vi "RealTimeAcq_SynthFoc.vi"(4 "Frames/s":sgl=2.0, 5 "return to start":bool, 6 "Scan Axis":i8=3, 7 "Motion Board ID":T3=1 min=1 max=32 step=1, 8 "BKPT Shift":i32=75, 9 "mode":T1=enum."Full 25 Ch") -> (0 "error out":errorcluster, 2 "Bd ID Out":T2)   [LabVIEW 2022 SP3]
uses:
  ScanningControl/Motion Controllers/-MotionRoutines/MotionGlobals.vi
  <vilib>/Motion/FlexMotion/FunctionsVIs/Trajectory.llb/Load Acceleration/Deceleration.flx
  <vilib>/Motion/FlexMotion/CustomControls/CustomControls.llb/Axis To Control.flx
  <vilib>/Motion/FlexMotion/CustomControls/CustomControls.llb/Program.flx
  <instrlib>/niScope/Acquire/Fetch/niScope Multi Fetch Binary 8.vi
  <vilib>/Platform/TimedLoop/XDataNode/XDataNode.xnode
  <vilib>/Platform/TimedLoop/XDataNode/nitl_modes.ctl
  <vilib>/Platform/TimedLoop/XDataNode/XDNodeRunTimeDep.lvlib
  <vilib>/Platform/TimedLoop/XDataNode/wakeup.ctl
  <vilib>/Platform/TimedLoop/XDataNode/timing_clust.ctl
  <vilib>/Motion/FlexMotion/FunctionsVIs/Trajectory.llb/Wait for Move Complete (8 axes).flx
  <instrlib>/Acqiris Dx/Acqiris Dx.lvlib
  <vilib>/DAQmx/write.llb/DAQmx Write (Digital 1D Bool NChan 1Samp 1Line).vi
  Real Time/-RT_support/RealTimeMode.ctl
  Annular Array/-SynthApperture/TimeShiftDataI8.vi
  <vilib>/Analysis/NI_AALBase.lvlib
  <vilib>/Analysis/baseanly.llb/Mean (DBL).vi
panel:
  in  "Velocity Scale (%)":i16(slide) scale=50.0..110.0
  in  "Raw Name":string="raw"
  in  "Save Raw":bool
  in  "Type of Mean":u16(ring) items=["Mean from lines", "Mean just lines", "Poly Mean", "No mean"]
  out "Display queue":i32
  out "SF queue":i32
  out "Record queue":i32
  out "Display index":i32
  out "Read Loop":i32
  out "Read Data index":i32
  in  "Round to ROC?":bool
  in  "F3 20 MHz":dbl[](array[numeric])=[0.0, 0.0021173000000000003, 0.002217038688303391, 0.003063649156506908, 0.0031631091439381287, 0.0038030513383040436, 0.003902223261134889, 0.004435332245982045, 0.004534208485358321, 0.004999044189180914]
  in  "F2 40MHz":sgl[](array[numeric])=[0.0, 0.00132, 0.00142, 0.0019, 0.002, 0.00236, 0.00245, 0.00275, 0.00285, 0.0031]
  in  "One Way Receive":bool
  out "SF Index":i32
  in  "stop out":bool
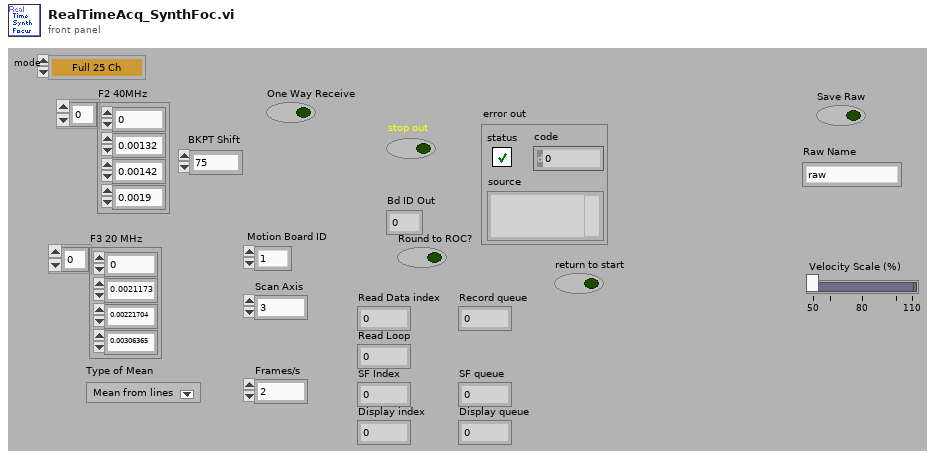
[diagram p1: front panel]
types:
  T1 = typedef "RealTimeMode.ctl" = enum16{"1T/5R", "1T/5R Deep Mem", "Full 25 Ch", "Drop Ch 5", "Drop Ch 5,4", "Drop Ch 5,4,3", "Drop Ch 5,4,3,2", "All 25 FIFO CH by CH", "Line by line 2 Ch", "Line by line All", "Deep Memory 2 CH", "Drop Ch 5 (3 Trig)", "test", "Drop Ch 5 XMIT", "Drop Ch 5,4 XMIT", "Drop Ch 5,4,3 XMIT"}
  T2 = typedef "Bd Id Out" = u8
  T3 = typedef "Board Id" = u8
  T4 = typedef "location.ctl" = enum16{"Automatic", "WCM Main", "Hawaii", "Columbia MM3000", "Columbia  NI System", "NYU", "RRI 2", "UHI Allen", "CUMC RT", "Chiba", "Stony Brook", "WCM Microscopy", "WCM Aeoretch", "WCM Optics Lab", "WCM Main 2Axis", "WCM Rotation", "WCM SAM SMAC", "SERI GP"}
  T5 = typedef "Program.flx" = u8
  T6 = typedef "XDNodeRunTimeDep.lvlib/timing_clust.ctl" = cluster{"Expected End [f-1]":u64, "Actual End [f-1]":u64, "Finished Late? [f-1]":bool, "Expected End [i-1]":u64, "Actual End [i-1]":u64, "Finished Late? [i-1]":bool, "Expected Start [i]":u64, "Actual Start [i]":u64, "Expected Start [f]":u64, "Actual Start [f]":u64, "Source Name":string, "Structure Name":string, "Period":i64, "Deadline":i64, "Offset":i64, "Start":i64, "Priority":i32, "Timeout":i32, "Mode":T7, "Wakeup Reason":T8, "Error":errorcluster, "Source Type":string, "Secondary Source Type":string, "Global End Time":u64, "Global Start Time":u64, "Frame Duration":u64, "Iteration Duration":u64, "Assigned CPU":i32, "I/O Scan Engine Mode":u32}
  T7 = typedef "XDNodeRunTimeDep.lvlib/nitl_modes.ctl" = enum32{"No Change", "Process missed periods, maintain original phase", "Discard missed periods, maintain original phase", "Process missed periods, ignore original phase", "Discard missed periods, ignore original phase"}
  T8 = typedef "XDNodeRunTimeDep.lvlib/wakeup.ctl" = enum32{"Normal", "Aborted", "Asynchronous wakeup", "Timing source error", "Timed loop error", "Timeout"}
  T9 = cluster{"gain":dbl, "wfm":i8[][], bool, "max queue size (-1, unlimited)":i32}
  T10 = typedef "Axis To Control.flx" = u16
  T11 = cluster{"ZoneStart":sgl[], "ZoneShift":sgl[], "ZoneLength":sgl[]}
  T12 = cluster{"ZoneStart":sgl[], "ZoneShift":sgl[], "ZoneLength":sgl[]}[][]
  T13 = cluster{"ZoneStart":sgl[], "ZoneShift":sgl[], "ZoneLength":sgl[]}[]
  T14 = cluster{"actualSamples":i32, "absoluteInitialX":dbl, "relativeInitialX":dbl, "xIncrement":dbl, "offset":dbl, "gain":dbl, "reserved1":dbl, "reserved2":dbl}[]
  T15 = cluster{"actualSamples":i32, "absoluteInitialX":dbl, "relativeInitialX":dbl, "xIncrement":dbl, "offset":dbl, "gain":dbl, "reserved1":dbl, "reserved2":dbl}
  T16 = cluster{"gain":dbl, "wfm":i8[][], "Reverse?":bool, i32}
  T17 = cluster{"dig gain":dbl, "Array":i8[][], "Reverse?":bool}
  T18 = typedef "Resource Out (Enum).flx" = u16
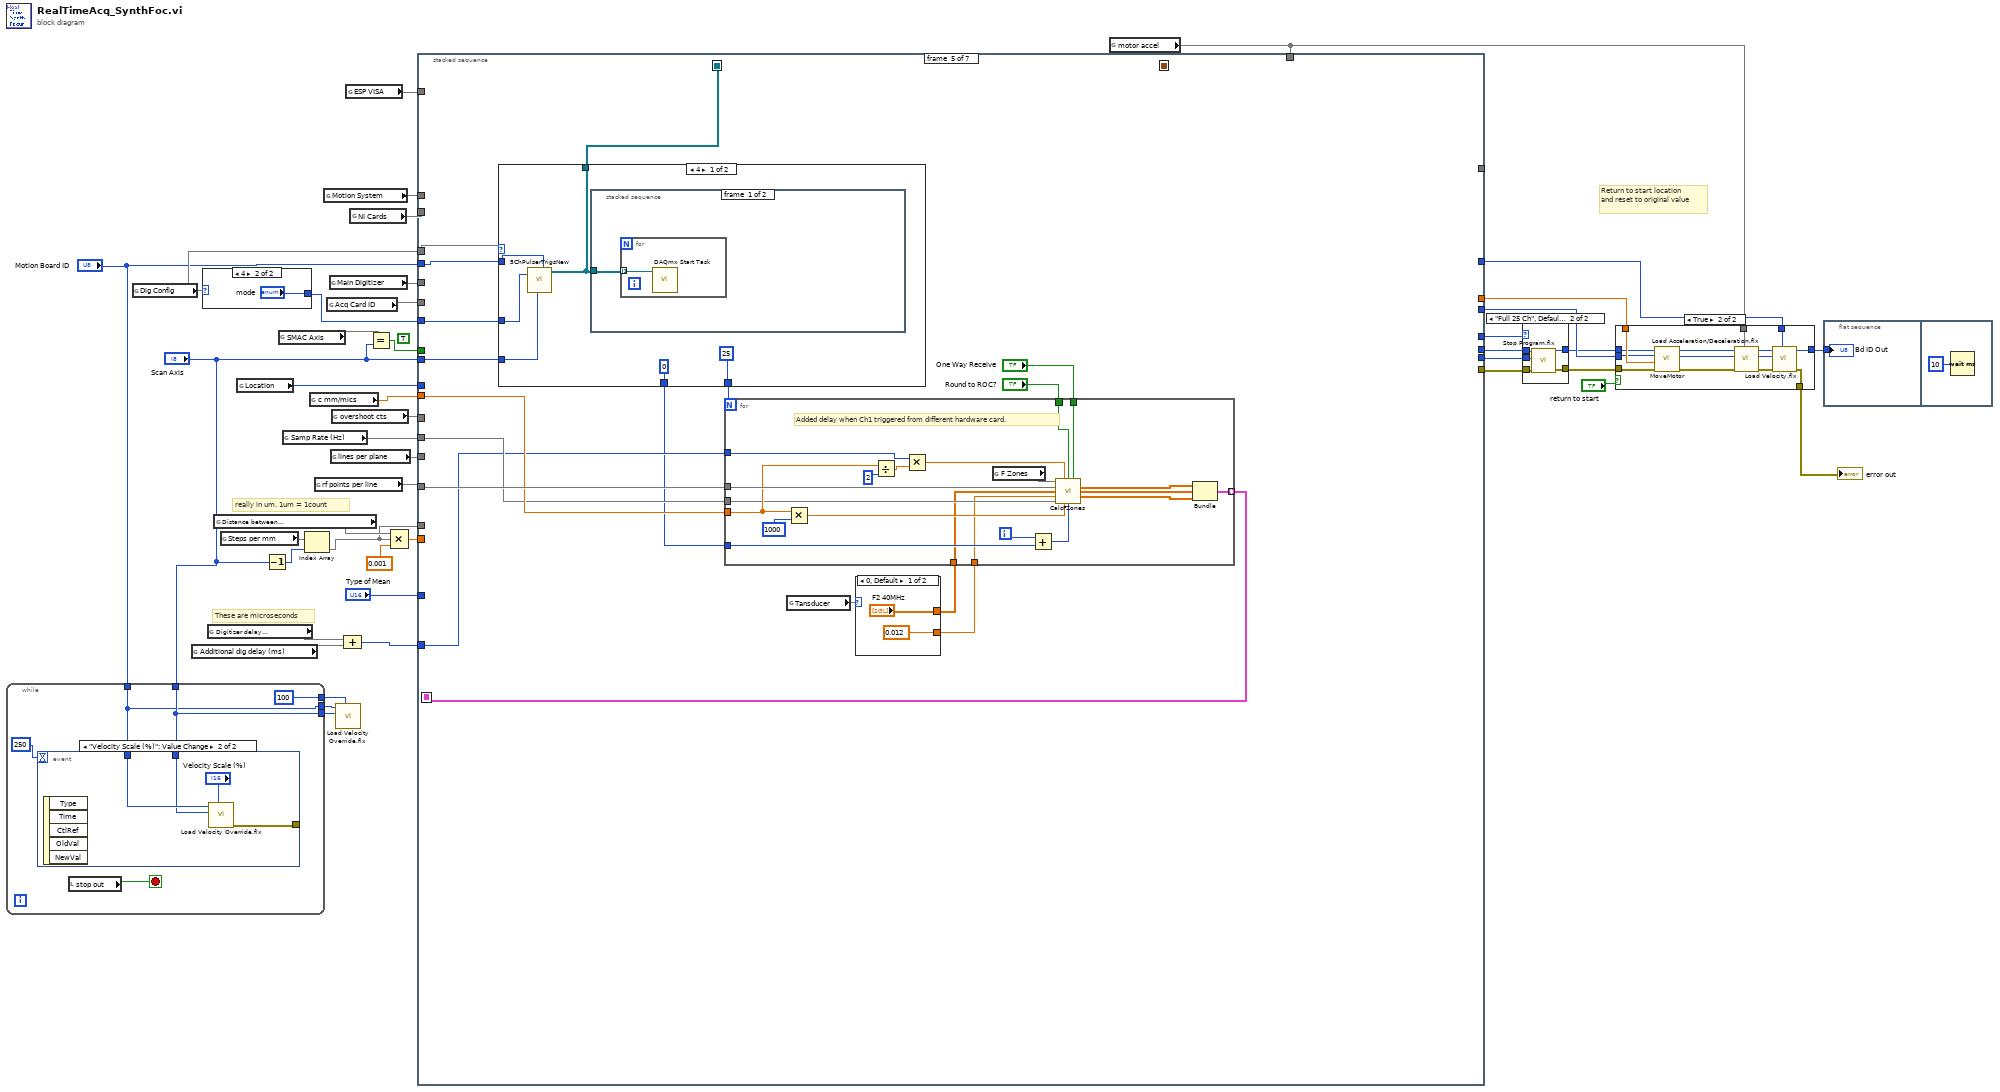
[diagram p0: block diagram]
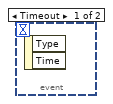
[diagram p2: hidden frame]
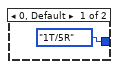
[diagram p3: hidden frame]
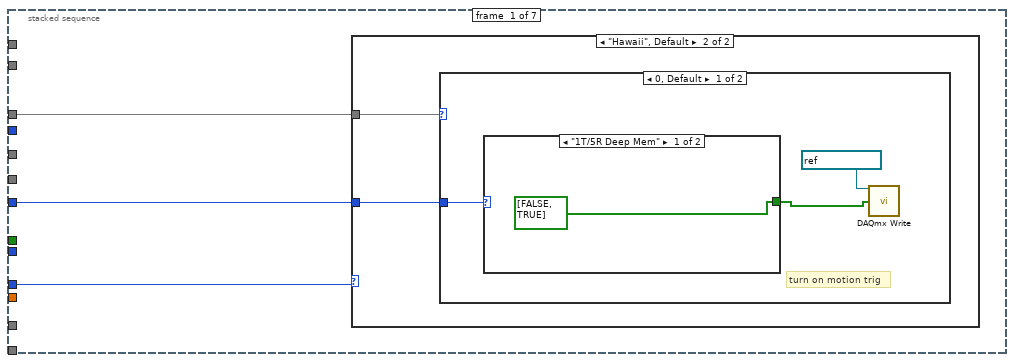
[diagram p6: hidden frame]
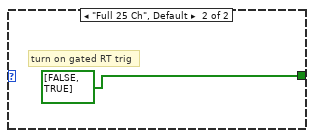
[diagram p8: hidden frame]
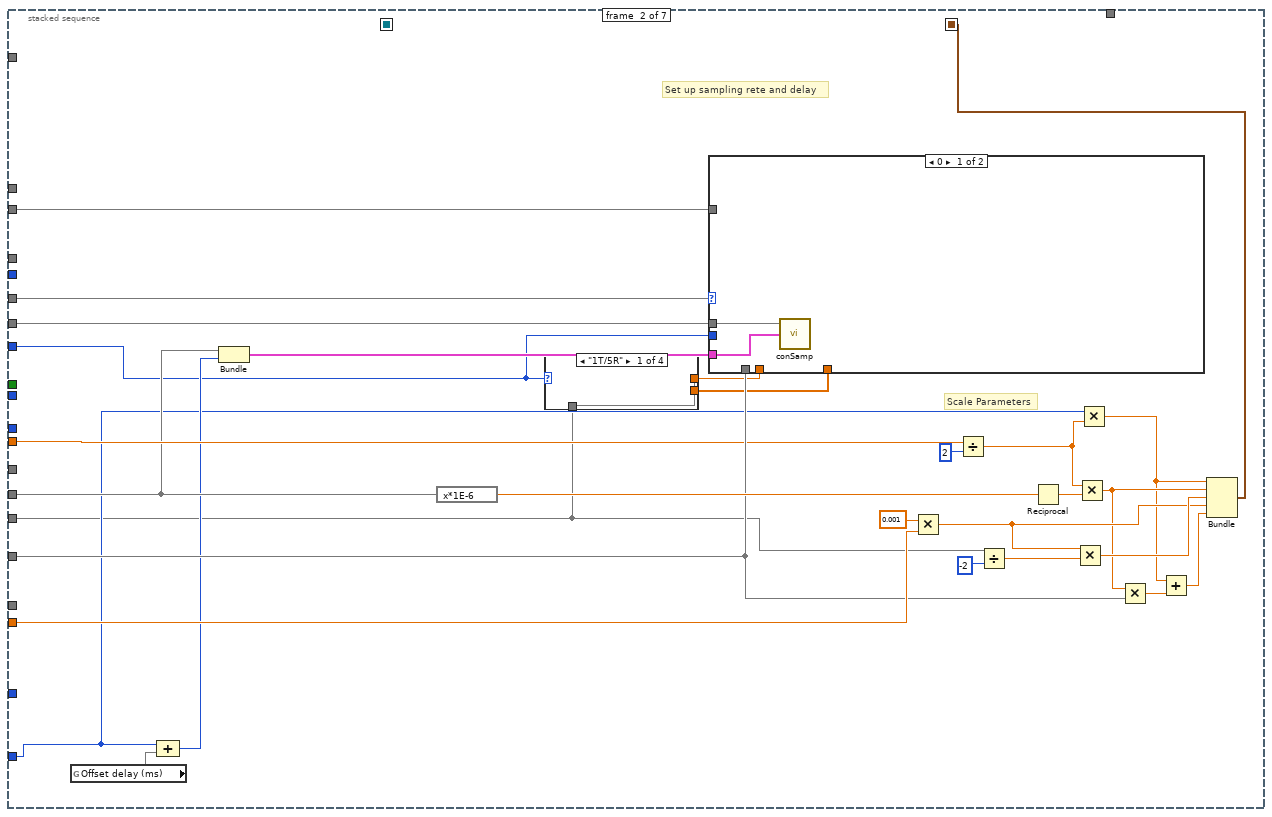
[diagram p10: hidden frame]
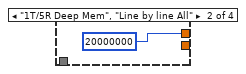
[diagram p11: hidden frame]
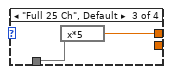
[diagram p12: hidden frame]
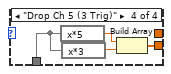
[diagram p13: hidden frame]
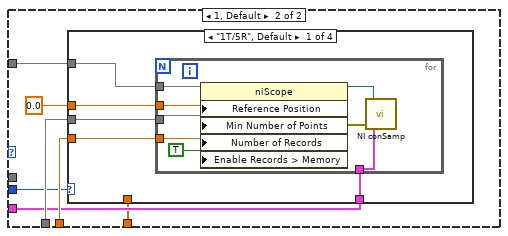
[diagram p14: hidden frame]
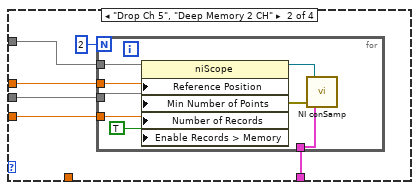
[diagram p15: hidden frame]
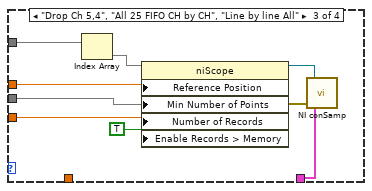
[diagram p16: hidden frame]
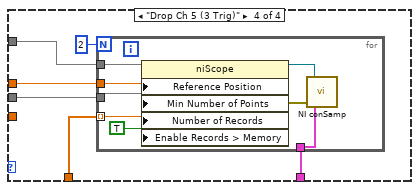
[diagram p17: hidden frame]
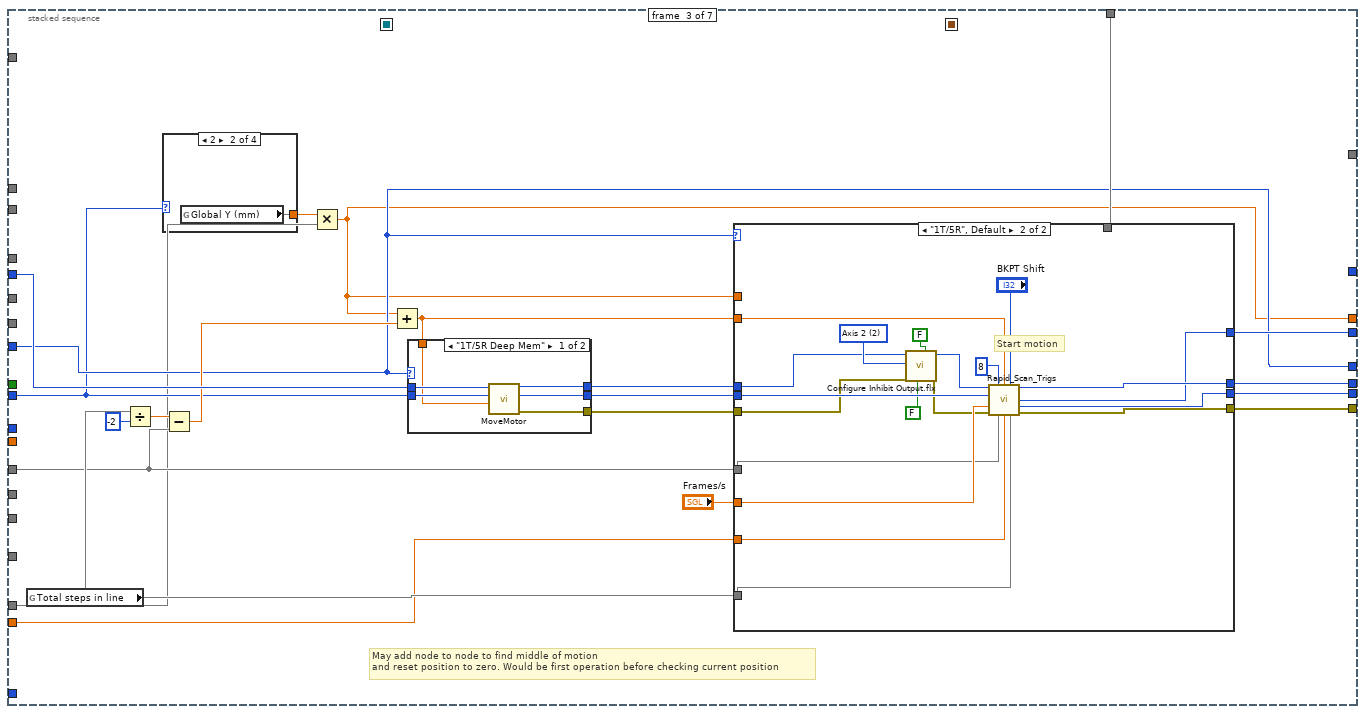
[diagram p18: hidden frame]
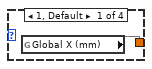
[diagram p19: hidden frame]
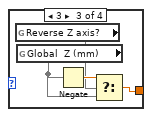
[diagram p20: hidden frame]
diagram:
  (unwired) TRUE
  # "These are microseconds"
  # "really in um. 1um = 1count"
  # "Return to start location and reset to original value"
  n1 = while {
    tunnel: "Motion Board ID" -> [w44]
    tunnel: "Scan Axis" -> [w45]
    tunnel: [100] -> w6
    tunnel: [w45] -> w5
    tunnel: [w44] -> w4
    stop <- w48 stop-if-true
    n2 = event shown="[1] \"Velocity Scale (%)\": Value Change" {
      selector: _ -> [_ _]
      dyn-events: _ -> [_ _]
      timeout: 250 -> [_ _]
      tunnel: w44 -> [_ w51]
      tunnel: w45 -> [_ w50]
      tunnel: [_ w49] -> _
      event Timeout {
        n3 = event-data() -> ()  [unwired: 1 in, 2 out]
      }
      event "Velocity Scale (%)": Value Change {
        n4 = event-data() -> ()  [unwired: 1 in, 5 out]
        n5 = call <vilib>:"Load Velocity Override.flx"("Override  Percentage (100%)"="Velocity Scale (%)", "Axis or Vector Space"=w50, "Board ID"=w51) -> ("error out"=w49:errorcluster)  [unwired: 4 in, 2 out]
      }
    }
    n6 = local read "stop out"() -> (w48:bool)
  }
  n7 = global read "MotionGlobals.vi" "Dig Config"() -> (w13)
  n8 = global read "MotionGlobals.vi" "Additional dig delay (ms)"() -> (w24)
  n9 = case shown="4" w13 {
    tunnel: [RealTimeMode."1T/5R" ("mode 2") "mode"] -> w15
    frame 0, Default {
    }
    frame 4 {
    }
  }
  n10 = global read "MotionGlobals.vi" "Digitizer delay\n (ms)"() -> (w25)
  n11 = global read "MotionGlobals.vi" "Distance between\nscan lines (mm)"() -> (w33)
  n12 = global read "MotionGlobals.vi" "Steps per mm"() -> (w12)
  n13 = global read "MotionGlobals.vi" "Location"() -> (w2:T4)
  n14 = Decrement(x="Scan Axis") -> (x-1=w11:i8)
  n15 = global read "MotionGlobals.vi" "SMAC Axis"() -> (w1)
  n16 = global read "MotionGlobals.vi" "Samp Rate (Hz)"() -> (w22)
  n17 = Index Array(array=w12, index=w11) -> (element=w10)
  n18 = global read "MotionGlobals.vi" "c mm/mics"() -> (w26:sgl)
  n19 = global read "MotionGlobals.vi" "rf points per line"() -> (w42)
  n20 = global read "MotionGlobals.vi" "Motion System"() -> (w9)
  n21 = global read "MotionGlobals.vi" "Acq Card ID"() -> (w30)
  n22 = global read "MotionGlobals.vi" "Main Digitizer"() -> (w31)
  n23 = global read "MotionGlobals.vi" "lines per plane"() -> (w43)
  n24 = global read "MotionGlobals.vi" "overshoot cts"() -> (w41)
  n25 = call <vilib>:"Load Velocity Override.flx"("Override  Percentage (100%)"=w6, "Axis or Vector Space"=w5, "Board ID"=w4) -> ()  [unwired: 4 in, 3 out]
  n26 = Compound Arithmetic op=ADD(w25, w24) -> (w23:i32)
  n27 = global read "MotionGlobals.vi" "ESP VISA"() -> (w16)
  n28 = global read "MotionGlobals.vi" "NI Cards"() -> (w3)
  n29 = Equal?(x=w1, y="Scan Axis") -> (x = y?=w21:bool)
  n30 = Compound Arithmetic op=MULTIPLY(w33, w10, 0.001) -> (w32:dbl)
  n31 = global read "MotionGlobals.vi" "motor accel"() -> (w28)
  n32 = stacked-sequence {
    seq-local: [_ w85 _ _ _ _ _] -> [_ _ _ _ _ w299 _]
    seq-local: [_ _ _ _ w242 _ _] -> [_ _ _ _ _ w298 _]
    seq-local: [_ _ _ _ w239 _ _] -> [_ _ _ _ _ _ w2097]
    tunnel: w30 -> [_ w92 _ _ _ w306 _]
    tunnel: w43 -> [_ w67 _ _ _ w305 _]
    tunnel: [_ _ w181 _ _ _ _] -> w37
    tunnel: [_ _ w180 _ _ _ _] -> w39
    tunnel: w42 -> [_ w75 _ _ w248 w304 _]
    tunnel: [_ _ w178 _ _ _ _] -> w38
    tunnel: [_ _ w165 _ _ _ _] -> w36
    tunnel: w41 -> [_ _ w174 _ _ _ _]
    tunnel: [_ _ w177 _ _ _ _] -> w40
    tunnel: "Motion Board ID" -> [_ _ w173 w229 w238 w303 _]
    tunnel: [_ _ w168 _ _ _ _] -> w35
    tunnel: w15 -> [w56 w66 w168 _ w236 w295 _]
    tunnel: "Scan Axis" -> [_ _ w167 _ w232 w296 _]
    tunnel: w32 -> [_ w78 w172 _ _ _ _]
    tunnel: w31 -> [_ w77 _ _ _ w302 _]
    tunnel: [_ _ _ _ _ w301 _] -> w29
    tunnel: w28 -> [_ _ w170 _ _ _ _]
    tunnel: w9 -> [_ _ _ w230 _ w300 _]
    tunnel: [_ _ _ _ _ w300 _] -> _
    tunnel: w2 -> [w57 _ _ _ _ _ w2099]
    tunnel: w26 -> [_ w74 _ _ w247 _ _]
    tunnel: w23 -> [_ w70 _ _ w245 _ _]
    tunnel: w22 -> [_ w73 _ _ w246 _ _]
    tunnel: w21 -> [_ _ _ _ _ w294 _]
    tunnel: w3 -> [_ w69 _ _ _ w297 _]
    tunnel: w16 -> [_ _ _ _ _ _ _]
    tunnel: "Type of Mean" -> [_ _ _ _ _ w293 _]
    tunnel: w13 -> [w55 _ _ _ w237 _ w2095]
    tunnel: w10 -> [_ _ w164 _ _ _ _]
    frame #0 {
      n33 = case shown="\"Hawaii\", Default" w57 {
        tunnel: w56 -> [_ w59]
        tunnel: w55 -> [_ w58]
        frame "UHI Allen", "CUMC RT" {
        }
        frame "Hawaii", Default {
          n34 = case shown="0, Default" w58 {
            tunnel: w59 -> [w62 _]
            frame 0, Default {
              # "turn on motion trig"
              n35 = case shown="\"1T/5R Deep Mem\"" w62 {
                tunnel: [bool[] [FALSE, TRUE] ("data") bool[] [FALSE, TRUE] ("data")] -> w60
                frame "1T/5R Deep Mem" {
                }
                frame "Full 25 Ch", Default {
                  # "turn on gated RT trig"
                }
              }
              n36 = call-poly <vilib>:"DAQmx Write.vi"("task/channels in"=refnum<k21> "DIO-L2 L3", "data"=w60) -> ()  [unwired: 11 in, 3 out]
            }
            frame 4 {
            }
          }
        }
      }
    }
    frame #1 {
      # "Scale Parameters"
      # "Set up sampling rete and delay"
      n37 = global read "MotionGlobals.vi" "Offset delay (ms)"() -> (w72)
      n38 = Compound Arithmetic op=ADD(w70, w72) -> (w71:i32)
      n39 = Bundle("Samp Rate (Hz)"=w73, w71) -> (w93:cluster{"Samp Rate (Hz)":void, i32})  [unwired: 1 out]
      n40 = expression code="x*1E-6"(w73) -> (w76:dbl)
      n41 = case shown="\"1T/5R\"" w66 {
        tunnel: [w94 20000000 w96 _] -> w68
        tunnel: w67 -> [w94 _ w97 w101]
        tunnel: [_ _ _ w98] -> w65
        frame "1T/5R" {
        }
        frame "1T/5R Deep Mem", "Line by line All" {
        }
        frame "Full 25 Ch", Default {
          n42 = expression code="x*5"(w97) -> (w96:dbl)
        }
        frame "Drop Ch 5 (3 Trig)" {
          n43 = expression code="x*5"(w101) -> (w100:dbl)
          n44 = expression code="x*3"(w101) -> (w99:dbl)
          n45 = Build Array(w100, w99) -> (w98:dbl[])
        }
      }
      n46 = case shown="0" w77 {
        tunnel: w93 -> [w103 w108]
        tunnel: w92 -> [w102 _]
        tunnel: w75 -> [_ w109]
        tunnel: w68 -> [_ w110]
        tunnel: w69 -> [_ w107]
        tunnel: w66 -> [_ w105]
        tunnel: w65 -> [_ w104]
        frame 0 {
          n47 = call "conSamp.vi"("Sampling"=w103, "InstrumentID"=w102) -> ()  [unwired: 1 in, 2 out]
        }
        frame 1, Default {
          n48 = case shown="\"1T/5R\", Default" w105 {
            tunnel: w110 -> [w115 w129 w146 _]
            tunnel: w109 -> [w114 w128 w145 w152]
            tunnel: w108 -> [w113 w127 w144 w151]
            tunnel: w107 -> [w112 w126 w142 w150]
            tunnel: 0.0 -> [w111 w125 w143 w149]
            tunnel: w104 -> [_ _ _ w147]
            frame "1T/5R", Default {
              n49 = for {
                tunnel: w115 -> [w118]
                tunnel: w114 -> [w123]
                tunnel: w112 -> [w120]
                tunnel: w113 -> [w119]
                tunnel: w111 -> [w117]
                n50 = property class="niScope"(reference=w120, "Reference Position"=w117, "Min Number of Points"=w123, "Number of Records"=w118, "Enable Records > Memory"=TRUE) -> (reference out=w122:refnum<k15>, error out=w121:errorcluster)  [unwired: 1 in]
                n51 = call "NI conSamp.vi"("error in"=w121, "Sampling"=w119, "InstrumentID"=w122) -> ()  [unwired: 2 out]
              }
            }
            frame "Drop Ch 5", "Deep Memory 2 CH" {
              n52 = for {
                N: 2 -> [_]
                tunnel: w129 -> [w132]
                tunnel: w128 -> [w137]
                tunnel: w126 -> [w134]
                tunnel: w127 -> [w133]
                tunnel: w125 -> [w131]
                n53 = property class="niScope"(reference=w134, "Reference Position"=w131, "Min Number of Points"=w137, "Number of Records"=w132, "Enable Records > Memory"=TRUE) -> (reference out=w136:refnum<k15>, error out=w135:errorcluster)  [unwired: 1 in]
                n54 = call "NI conSamp.vi"("error in"=w135, "Sampling"=w133, "InstrumentID"=w136) -> ()  [unwired: 2 out]
              }
            }
            frame "Drop Ch 5,4", "All 25 FIFO CH by CH", "Line by line All" {
              n55 = Index Array(array=w142) -> (element=w138)  [unwired: 1 in]
              n56 = property class="niScope"(reference=w138, "Reference Position"=w143, "Min Number of Points"=w145, "Number of Records"=w146, "Enable Records > Memory"=TRUE) -> (reference out=w141:refnum<k15>, error out=w140:errorcluster)  [unwired: 1 in]
              n57 = call "NI conSamp.vi"("error in"=w140, "Sampling"=w144, "InstrumentID"=w141) -> ()  [unwired: 2 out]
            }
            frame "Drop Ch 5 (3 Trig)" {
              n58 = for {
                N: 2 -> [_]
                tunnel: w147 -> [w155] mode=indexing
                tunnel: w152 -> [w160]
                tunnel: w150 -> [w157]
                tunnel: w151 -> [w156]
                tunnel: w149 -> [w154]
                n59 = property class="niScope"(reference=w157, "Reference Position"=w154, "Min Number of Points"=w160, "Number of Records"=w155, "Enable Records > Memory"=TRUE) -> (reference out=w159:refnum<k15>, error out=w158:errorcluster)  [unwired: 1 in]
                n60 = call "NI conSamp.vi"("error in"=w158, "Sampling"=w156, "InstrumentID"=w159) -> ()  [unwired: 2 out]
              }
            }
          }
        }
      }
      n61 = Multiply(x=0.001, y=w78) -> (x*y=w83:dbl)
      n62 = Divide(x=w74, y=2) -> (x/y=w86:sgl)
      n63 = Divide(x=w67, y=-2) -> (x/y=w88:dbl)
      n64 = Reciprocal(x=w76) -> (1/x=w91:dbl)
      n65 = Multiply(x=w83, y=w88) -> (x*y=w84:dbl)
      n66 = Multiply(x=w86, y=w91) -> (x*y=w82:dbl)
      n67 = Multiply(x=w70, y=w86) -> (x*y=w80:sgl)
      n68 = Multiply(x=w82, y=w75) -> (x*y=w81:dbl)
      n69 = Add(x=w80, y=w81) -> (x+y=w79:sgl)
      n70 = Bundle(w80, w82, w84, w83, w79) -> (w85:cluster{sgl, dbl, dbl, dbl, sgl})  [unwired: 1 out]
    }
    frame #2 {
      # "May add node to node to find middle of motion\nand reset position to zero. Would be first operation before checking current position"
      n71 = global read "MotionGlobals.vi" "Total steps in line"() -> (w176)
      n72 = Divide(x=w176, y=-2) -> (x/y=w175:dbl)
      n73 = case shown="2" w167 {
        tunnel: [w183 w184 w185 w189] -> w166
        frame 1, Default {
          n74 = global read "MotionGlobals.vi" "Global X (mm)"() -> (w183)
        }
        frame 2 {
          n75 = global read "MotionGlobals.vi" "Global Y (mm)"() -> (w184)
        }
        frame 3 {
          n76 = global read "MotionGlobals.vi" "Reverse Z axis?"() -> (w186)
          n77 = global read "MotionGlobals.vi" "Global  Z (mm)"() -> (w187)
          n78 = Negate(x=w187) -> (-x=w188:dbl)
          n79 = Select(t=w188, s=w186, f=w187) -> (s? t:f=w185:dbl)
        }
        frame 4 {
          n80 = global read "MotionGlobals.vi" "Global  Axis 4"() -> (w189)
        }
      }
      n81 = Subtract(x=w175, y=w174) -> (x-y=w171:dbl)
      n82 = Multiply(x=w166, y=w164) -> (x*y=w165:dbl)
      n83 = Add(x=w165, y=w171) -> (x+y=w169:dbl)
      n84 = case shown="\"1T/5R Deep Mem\"" w168 {
        tunnel: w173 -> [w195 w197]
        tunnel: w167 -> [w194 w196]
        tunnel: [w193 w197] -> w161
        tunnel: [w192 w196] -> w163
        tunnel: [w191 _] -> w162
        tunnel: w169 -> [w190 _]
        frame "1T/5R Deep Mem" {
          n85 = call "MoveMotor.vi"("Target Position (0)"=w190, "Axis or Vector Space"=w194, "Motion Bd ID"=w195) -> ("error out"=w191:errorcluster, "Resource Output"=w192:u16, "Bd ID Out"=w193:u8)  [unwired: 2 in, 4 out]
        }
        frame "Full 25 Ch", Default {
        }
      }
      n86 = case shown="\"1T/5R\", Default" w168 {
        tunnel: "Frames/s" -> [w207 w228]
        tunnel: [w198 w227] -> w181
        tunnel: [w209 w226] -> w180
        tunnel: [_ w225] -> w178
        tunnel: [w208 w224] -> w177
        tunnel: w176 -> [w205 w223]
        tunnel: w172 -> [_ w222]
        tunnel: w174 -> [_ w221]
        tunnel: w161 -> [w209 w211]
        tunnel: w163 -> [w208 w220]
        tunnel: w162 -> [w199 w210]
        tunnel: w169 -> [_ w219]
        tunnel: w165 -> [w206 _]
        tunnel: w170 -> [_ _]
        frame "1T/5R Deep Mem", "Line by line All" {
          w201 = T5 6 ("Program (1)")
          w204 = FALSE
          n87 = call "Modulo_Triggers.vi"("Motion Settings In"=w209, "Axis"=w208, "Reverse ?"=w204, "Program (1)"=w201, 7:w207, "error in (no error)"=w199, 12:w205, "Offset"=w206) -> ("error out"=w200:errorcluster)  [unwired: 1 in, 6 out]
          n88 = Increment(x=w201) -> (x+1=w202:T5)
          n89 = Not(x=w204) -> (.not. x?=w203:bool)
          n90 = call "Modulo_Triggers.vi"("Motion Settings In"=w209, "Axis"=w208, "Reverse ?"=w203, "Program (1)"=w202, 7:w207, "error in (no error)"=w200, 12:w205, "Offset"=w206) -> ("error out"=w198:errorcluster)  [unwired: 1 in, 6 out]
        }
        frame "1T/5R", Default {
          w214 = T10 2 items=["Axis 1"=1, "Axis 2"=2, "Axis 3"=3, "Axis 4"=4, "Axis 5"=5, "Axis 6"=6, "Axis 7"=7, "Axis 8"=8] ("Axis")
          # "Start motion"
          n91 = call <vilib>:"Configure Inhibit Output.flx"("Enable"=FALSE, "Polarity (Active Low)"=FALSE, "error in (no error)"=w210, "Axis"=w214, "Board ID"=w211) -> ("error out"=w217:errorcluster, "Bd ID Out"=w218:T2)  [unwired: 1 in, 4 out]
          n92 = call "Rapid_Scan_Trigs.vi"("Board ID"=w218, "Program (1)"=T5 8, "Start Position"=w219, "BKPT Shift"="BKPT Shift", "Scan Axis"=w220, "# frames/ s"=w228, "error in (no error)"=w217, "overshoot"=w221, "step interval"=w222, "Total Steps (one way)"=w223) -> ("Bd ID Out"=w226:u8, "Axis Resource out"=w224:u16, "Program ID"=w225:u8, "error out"=w227:errorcluster)  [unwired: 1 in, 1 out]
        }
      }
    }
    frame #3 {
      n93 = case shown="0, Default" w230 {
        tunnel: w229 -> [w231 _]
        frame 0, Default {
          n94 = call "CheckLimStat.vi"("Motion Board ID"=w231) -> ()
        }
        frame 1, 7 {
        }
      }
    }
    frame #4 {
      n95 = case shown="4" w237 {
        tunnel: [25 5] -> w241
        tunnel: [u32 0 w267] -> w240
        tunnel: [w253 _] -> w239
        tunnel: w238 -> [w256 _]
        tunnel: w236 -> [w255 _]
        tunnel: w232 -> [w254 _]
        frame 4 {
          n96 = call "5ChPulserTrigsNew.vi"("Motion Settings"=w256, "Digitizer Settings"=w255, "Axis"=w254) -> ("5CH Pulser Tasks"=w253:refnum<k21>[])  [unwired: 6 in, 1 out]
          n97 = stacked-sequence {
            tunnel: w253 -> [w259 _]
            frame #0 {
              n98 = for {
                tunnel: w259 -> [w260] mode=indexing
                n99 = call <vilib>:"DAQmx Start Task.vi"("task/channels in"=w260) -> ()  [unwired: 1 in, 14 out]
              }
            }
            frame #1 {
              n100 = for {
                tunnel: bool[][] [[TRUE], [FALSE]] ("data") -> [w262] mode=indexing
                n101 = flat-sequence {
                  tunnel: w262 -> [w265]
                  tunnel: [w265] -> w263
                  tunnel: w263 -> [w266]
                  frame #0 {
                    n102 = Wait (ms)(milliseconds to wait=u32 25) -> ()  [unwired: 1 out]
                  }
                  frame #1 {
                    n103 = call "DAQ Assistant"("data"=w266) -> ()  [unwired: 17 in, 2 out]
                  }
                }
              }
            }
          }
        }
        frame 0, Default {
          n104 = global read "MotionGlobals.vi" "Switch T/R"() -> (w270)
          n105 = Decrement(x=w270) -> (x-1=w269:dbl)
          n106 = Multiply(x=w269, y=5) -> (x*y=w267:i32)
        }
      }
      n107 = global read "MotionGlobals.vi" "Tansducer"() -> (w235)
      n108 = case shown="0, Default" w235 {
        tunnel: ["F2 40MHz" "F3 20 MHz"] -> w234
        tunnel: [0.012 ("ROC (mm)") 0.031 ("ROC (mm)")] -> w233
        frame 0, Default {
        }
        frame 1 {
        }
      }
      n109 = for {
        N: w241 -> [_]
        tunnel: w248 -> [w288]
        tunnel: w247 -> [w281]
        tunnel: w246 -> [w276]
        tunnel: w245 -> [w287]
        tunnel: "One Way Receive" -> [w286]
        tunnel: "Round to ROC?" -> [w285]
        tunnel: [w283] -> w242 mode=indexing
        tunnel: w240 -> [w278]
        tunnel: w234 -> [w273]
        tunnel: w233 -> [w272]
        i -> [w277]
        # "Added delay when Ch1 triggered from different hardware card."
        n110 = Multiply(x=w281, y=1000) -> (x*y=w282:sgl)
        n111 = Divide(x=w281, y=2) -> (x/y=w291:sgl)
        n112 = Multiply(x=w287, y=w291) -> (x*y=w280:sgl)
        n113 = global read "MotionGlobals.vi" "F Zones"() -> (w290)
        n114 = Add(x=w277, y=w278) -> (x+y=w279:u32)
        n115 = call "CalcFZones.vi"("F- zones"=w290, "delay (mm)"=w280, "Round to ROC?"=w285, "One Way Receive"=w286, "# rf points per line"=w288, "Radii (m)"=w273, "ROC (m)"=w272, "Sampling Rate"=w276, "c (m/s)"=w282, "File index number"=w279) -> ("ZoneStart"=w275:sgl[], "ZoneShift"=w274:sgl[], "ZoneLength"=w284:sgl[])  [unwired: 3 out]
        n116 = Bundle("ZoneStart"=w275, "ZoneShift"=w274, "ZoneLength"=w284) -> (w283:T11)  [unwired: 1 in]
      }
    }
    frame #5 {
      n117 = case shown="True" w294 {
        tunnel: w306 -> [w315 _]
        tunnel: w305 -> [w316 w408]
        tunnel: w304 -> [w317 w407]
        tunnel: w303 -> [w313 w409]
        tunnel: w299 -> [w312 w406]
        tunnel: w302 -> [w311 _]
        tunnel: [w310 w410] -> w301
        tunnel: w300 -> [w309 _]
        tunnel: w298 -> [_ w405]
        tunnel: w295 -> [_ w404]
        tunnel: w297 -> [w308 w403]
        tunnel: w296 -> [_ w402]
        tunnel: w293 -> [_ w401]
        frame False {
          n118 = Index Array(array=w308) -> (element=w307)  [unwired: 1 in]
          n119 = while {
            tunnel: w317 -> [w339]
            tunnel: w316 -> [w329]
            tunnel: w315 -> [w338]
            shift-right: [w337] -> _
            shift-left: TRUE -> [w322]
            tunnel: w313 -> [w336]
            tunnel: w312 -> [w332]
            tunnel: w311 -> [w330]
            tunnel: w309 -> [w323]
            tunnel: w307 -> [w318]
            i -> [w331]
            stop <- w335 stop-if-true
            # "Display data"
            # "Get data"
            # "This is slower version for heavier mass motors. Scan stop, read data, scan etc"
            n120 = Select(t="1", s=w322, f="2") -> (s? t:f=w319:string)
            n121 = Select(t=T5 6 ("Program (1)"), s=w322, f=T5 7 ("Program (1)")) -> (s? t:f=w326:T5)
            n122 = case shown="0" w330 {
              tunnel: w339 -> [w349 w377]
              tunnel: w329 -> [w348 w376]
              tunnel: w338 -> [w362 _]
              tunnel: w336 -> [w361 w388]
              tunnel: [w360 w387] -> w334
              tunnel: w326 -> [w356 w386]
              tunnel: [w343 w378] -> w328
              tunnel: w318 -> [_ w380]
              tunnel: w322 -> [w345 w371]
              tunnel: [w346 w370] -> w327
              tunnel: w323 -> [_ _]
              tunnel: w319 -> [_ _]
              frame 0 {
                n123 = call <instrlib>:"Configure Memory Settings.vi"("Number of Samples (1000)"=w349, "Number of Segments (1)"=w348, "Instrument ID"=w362) -> ("error out"=w359:errorcluster, "dup Instrument ID"=w357:u32)  [unwired: 1 in, 2 out]
                n124 = call <instrlib>:"Start Acquisition.vi"("error in (no error)"=w359, "Instrument ID"=w357) -> ("error out"=w355:errorcluster, "dup Instrument ID"=w358:u32)  [unwired: 2 in]
                n125 = stacked-sequence {
                  tunnel: w355 -> [w369]
                  tunnel: [w369] -> w354
                  frame #0 {
                    n126 = Wait (ms)(milliseconds to wait=20) -> ()  [unwired: 1 out]
                  }
                }
                n127 = call <vilib>:"Run Program.flx"("error in (no error)"=w354, "Program (1)"=w356, "Board ID"=w361) -> ("error out"=w353:errorcluster, "Bd ID Out"=w360:T2)  [unwired: 4 out]
                n128 = stacked-sequence {
                  tunnel: w353 -> [w366]
                  tunnel: [w366] -> w352
                  frame #0 {
                    n129 = Wait (ms)(milliseconds to wait=20) -> ()  [unwired: 1 out]
                  }
                }
                n130 = call "WaitForSegs.vi"("Acqiris ID"=w358, "lines per plane"=w348, "error in"=w352, "Timeout"=5000) -> ("dup Instrument ID"=w351:u32, "error out"=w350:errorcluster)  [unwired: 2 out]
                n131 = call "GetWaveform.vi"("Acq ID Out"=w351, "Num Samps"=w349, "Num Segs"=w348, "error in"=w350) -> ("Acquired Waveform16 bit"=w347:i16[][], "error out"=w343:errorcluster)  [unwired: 2 in, 8 out]
                n132 = case shown="True" w345 {
                  tunnel: w347 -> [w363 w365]
                  tunnel: [w363 w364] -> w346
                  frame False {
                  }
                  frame True {
                    n133 = call "ReverseData.vi"("Array in"=w365) -> ("Array out"=w364:i16[][])
                  }
                }
              }
              frame 1, Default {
                w374 = u16 1 items=["Simple Read", "RT Read", "RT Save", "Scaled Voltage"] ("Read Method")
                n134 = property class="niScope"(reference=w380, "Number of Records"=w376, "Min Number of Points"=w377) -> (reference out=w382:refnum<k15>, error out=w381:errorcluster)  [unwired: 1 in]
                n135 = call <instrlib>:"niScope Initiate Acquisition.vi"("instrument handle"=w382, "error in"=w381) -> ("instrument handle out"=w375:refnum<k15>, "error out"=w385:errorcluster)  [unwired: 1 in, 11 out]
                n136 = stacked-sequence {
                  tunnel: w385 -> [w392]
                  tunnel: [w392] -> w384
                  frame #0 {
                    n137 = Wait (ms)(milliseconds to wait=u32 5) -> ()  [unwired: 1 out]
                  }
                }
                n138 = call <vilib>:"Run Program.flx"("error in (no error)"=w384, "Program (1)"=w386, "Board ID"=w388) -> ("error out"=w383:errorcluster, "Bd ID Out"=w387:T2)  [unwired: 4 out]
                n139 = stacked-sequence {
                  tunnel: w383 -> [w389]
                  tunnel: [w389] -> w379
                  frame #0 {
                    n140 = Wait (ms)(milliseconds to wait=u32 20) -> ()  [unwired: 1 out]
                  }
                }
                n141 = call "NI GetWaveform.vi"("Acq ID In"=w375, "Read Method"=w374, "timeout"=5.0, "Num Samps"=w377, "Reverse?"=w371, "Num Segs"=w376, "error in"=w379, "Channel"=1) -> ("Acquired Waveform16 bit"=w370:i8[][], "error out"=w378:errorcluster)  [unwired: 2 in, 4 out]
              }
            }
            n142 = case shown="No Error" w328 {
              selector: w328 -> [w394 w399]
              tunnel: [w395 w399] -> w333
              tunnel: [w398 TRUE] -> w335
              tunnel: w332 -> [w397 _]
              tunnel: w331 -> [w396 _]
              tunnel: w327 -> [w393 _]
              frame No Error {
                n143 = call "CurrentPlane.vi"("Axis Vals"=w397, "error in"=w394, "Frame"=w396, "Data"=w393) -> ("error out"=w395:errorcluster, "stop out"=w398:bool)  [unwired: 6 in]
              }
              frame Error {
              }
            }
            n144 = local write "SF Index"(w331) -> ()
            n145 = case shown="1, Default" w323 {
              tunnel: w334 -> [_ w342]
              tunnel: w333 -> [_ w341]
              tunnel: w326 -> [_ w340]
              frame 7 {
              }
              frame 1, Default {
                n146 = call <vilib>:"Stop Program.flx"("error in (no error)"=w341, "Program (1)"=w340, "Board ID"=w342) -> ()  [unwired: 6 out]
              }
            }
            n147 = Not(x=w322) -> (.not. x?=w337:bool)
          }
          n148 = global read "MotionGlobals.vi" "motor velocity"() -> (w310)
        }
        frame True {
          n149 = case shown="\"1T/5R Deep Mem\"" w404 {
            tunnel: [40000 40000 40000 40000 40000 40000 40000 40000 40000 40000 40000] -> w410
            tunnel: w409 -> [w436 w586 w744 w930 w1111 w1286 w1400 w1563 w1648 w1768 w1938]
            tunnel: w408 -> [w435 w582 w748 w912 w1093 w1282 w1404 w1564 w1649 w1734 w1917]
            tunnel: w407 -> [w434 w583 w726 w914 w1095 w1273 w1397 w1551 w1662 w1737 w1922]
            tunnel: w406 -> [w413 w551 w750 w935 w1116 w1291 w1406 w1569 w1656 w1754 w1943]
            tunnel: w405 -> [w429 w577 w758 w943 w1124 w1299 w1415 w1554 w1650 w1743 w1951]
            tunnel: w403 -> [w422 w560 w720 w906 w1084 w1271 w1390 w1549 w1643 w1726 w1912]
            tunnel: w402 -> [_ w562 _ _ _ _ _ _ _ w1761 _]
            tunnel: w401 -> [_ _ _ _ _ _ _ _ _ _ _]
            frame "1T/5R", Default {
              # "1T/5R flip flop version"
              n150 = Array To Cluster(array=w422) -> (cluster=w421:cluster{"[0]":void, "[1]":void, "[2]":void})
              n151 = Unbundle(w421) -> ("[0]"=w412, "[1]"=w420, "[2]"=w419)
              n152 = Obtain Queue(max queue size (-1, unlimited)=2, element data type=cluster{"gain":dbl, bool} {"gain"=0.0, TRUE}) -> (queue out=w444:refnum<queue>)  [unwired: 2 in, 3 out]
              n153 = Index Array(array=w429) -> (element=w426:T11)  [unwired: 1 in]
              n154 = Index Array(array=w429, index=1) -> (element=w425:T11)
              n155 = Index Array(array=w429, index=2) -> (element=w424:T11)
              n156 = Index Array(array=w429, index=3) -> (element=w427:T11)
              n157 = Index Array(array=w429, index=4) -> (element=w428:T11)
              n158 = Obtain Queue(max queue size (-1, unlimited)=5, element data type=i8[][] [] ("Array")) -> (queue out=w437:refnum<queue>)  [unwired: 2 in, 3 out]
              n159 = Obtain Queue(max queue size (-1, unlimited)=2, element data type=cluster{bool, "Array":i16[][]} {TRUE, "Array"=[]}) -> (queue out=w417:refnum<queue>)  [unwired: 3 in, 2 out]
              n160 = while {
                tunnel: w444 -> [w473]
                tunnel: [w504] -> w442
                tunnel: [w482] -> w441
                tunnel: w437 -> [w474]
                tunnel: w428 -> [w495]
                tunnel: w427 -> [w494]
                tunnel: w426 -> [w493]
                tunnel: w425 -> [w492]
                tunnel: w424 -> [w491]
                tunnel: [w469] -> w423
                tunnel: w417 -> [w486]
                i -> [w483]
                stop <- w504 stop-if-true
                w479 = 5000 ("timeout in ms (-1)")
                # "Dequeue data and synth focus"
                n161 = Dequeue Element(queue=w473, timeout in ms (-1)=w479) -> (queue out=w482:refnum<queue>, element=w503:cluster{"gain":dbl, bool}, error out=w481:errorcluster)  [unwired: 1 in, 1 out]
                n162 = Dequeue Element(queue=w474, timeout in ms (-1)=w479, error in (no error)=w481) -> (queue out=w472:refnum<queue>, element=w480:i8[][], error out=w478:errorcluster)  [unwired: 1 out]
                n163 = Unbundle(w503) -> (w485:bool)  [unwired: 1 out]
                n164 = call-poly "TimeShiftDataPoly.vi"("output cluster"=w493, "Array In"=w480) -> ("Array Out"=w466:i8[][])  [unwired: 1 in, 1 out]
                n165 = Dequeue Element(queue=w472, timeout in ms (-1)=w479, error in (no error)=w478) -> (queue out=w502:refnum<queue>, element=w499:i8[][], error out=w477:errorcluster)  [unwired: 1 out]
                n166 = call-poly "TimeShiftDataPoly.vi"("output cluster"=w492, "Array In"=w499) -> ("Array Out"=w490:i8[][])  [unwired: 1 in, 1 out]
                n167 = Dequeue Element(queue=w502, timeout in ms (-1)=w479, error in (no error)=w477) -> (queue out=w501:refnum<queue>, element=w498:i8[][], error out=w476:errorcluster)  [unwired: 1 out]
                n168 = call-poly "TimeShiftDataPoly.vi"("output cluster"=w491, "Array In"=w498) -> ("Array Out"=w489:i8[][])  [unwired: 1 in, 1 out]
                n169 = Dequeue Element(queue=w501, timeout in ms (-1)=w479, error in (no error)=w476) -> (queue out=w500:refnum<queue>, element=w497:i8[][], error out=w475:errorcluster)  [unwired: 1 out]
                n170 = call-poly "TimeShiftDataPoly.vi"("output cluster"=w494, "Array In"=w497) -> ("Array Out"=w488:i8[][])  [unwired: 1 in, 1 out]
                n171 = Dequeue Element(queue=w500, timeout in ms (-1)=w479, error in (no error)=w475) -> (queue out=w470:refnum<queue>, element=w496:i8[][], error out=w471:errorcluster)  [unwired: 1 out]
                n172 = call-poly "TimeShiftDataPoly.vi"("output cluster"=w495, "Array In"=w496) -> ("Array Out"=w487:i8[][])  [unwired: 1 in, 1 out]
                n173 = Get Queue Status(queue=w470, error in (no error)=w471) -> (queue out=w469:refnum<queue>, # elements in queue=w468:i32)  [unwired: 1 in, 6 out]
                n174 = Compound Arithmetic op=ADD(w490, w489, w488, w487) -> (w467:i8[][])
                n175 = expression code="x*2"(w467) -> (w465:i8[][])
                n176 = Multiply(x=w466, y=w465) -> (x*y=w464:i8[][])
                n177 = local write "SF queue"(w468) -> ()
                n178 = local read "stop out"() -> (w504:bool)
                n179 = Bundle(w485, w464) -> (w484:cluster{bool, i8[][]})  [unwired: 1 in]
                n180 = Lossy Enqueue Element(queue=w486, element=w484) -> ()  [unwired: 1 in, 4 out]
                "SF Index" <- w483
              }
              n181 = while {
                tunnel: [w449] -> w415
                tunnel: w417 -> [w451]
                tunnel: w413 -> [w456]
                tunnel: u16 13 ("bits A/D") -> [w447]
                i -> [w452]
                stop <- w457 stop-if-true
                # "Log compress and display data"
                n182 = Dequeue Element(queue=w451, timeout in ms (-1)=5000) -> (queue out=w450:refnum<queue>, element=w455:cluster{bool, "Array":i16[][]})  [unwired: 1 in, 2 out]
                n183 = Get Queue Status(queue=w450) -> (queue out=w449:refnum<queue>, # elements in queue=→"Display queue":i32)  [unwired: 2 in, 6 out]
                n184 = Unbundle(w455) -> (w454:bool, "Array"=w453:i16[][])
                n185 = case shown="True" w454 {
                  tunnel: [w461 w463] -> w459
                  tunnel: w453 -> [w461 w462]
                  frame False {
                  }
                  frame True {
                    n186 = call "ReverseData.vi"("Array in"=w462) -> ("Array out"=w463:i16[][])
                  }
                }
                n187 = Increment(x=w452) -> (x+1=w460:i32)
                n188 = call "CurrentPlane.vi"("bits A/D"=w447, "Axis Vals"=w456, "Frame"=w460, "Data"=w459) -> ("stop out"=w457:bool)  [unwired: 6 in, 1 out]
                n189 = local write "stop out"(w457) -> ()
                "Display index" <- w452
              }
              n190 = while {
                tunnel: w435 -> [_]
                tunnel: w434 -> [w530]
                tunnel: w436 -> [w537]
                tunnel: w444 -> [w536]
                tunnel: ["stop out"] -> w443
                tunnel: w412 -> [w506]
                tunnel: w437 -> [w515]
                tunnel: w420 -> [w518]
                tunnel: w419 -> [w517]
                i -> [w519]
                stop <- "stop out" stop-if-true
                # "Get next available frame and queue data"
                n191 = call <instrlib>:"niScope Initiate Acquisition.vi"("instrument handle"=w518) -> ("instrument handle out"=w521:refnum<k15>, "error out"=w522:errorcluster)  [unwired: 2 in, 11 out]
                n192 = call <instrlib>:"niScope Initiate Acquisition.vi"("instrument handle"=w517, "error in"=w522) -> ("instrument handle out"=w520:refnum<k15>, "error out"=w531:errorcluster)  [unwired: 1 in, 11 out]
                n193 = call "Rapid Read_NI.vi"("NI Card"=w506, "Channel"="0", "Motion Board ID"=w537, "rf points per line"=w530, "error in"=w531) -> ("dig gain"=w533:dbl, "Array"=w513:i8[][], "Reverse?"=w505:bool, "error out"=w508:errorcluster)  [unwired: 7 in]
                n194 = Bundle("dig gain"=w533, "Reverse?"=w505) -> (w534:cluster{"dig gain":dbl, "Reverse?":bool})  [unwired: 1 out]
                n195 = Lossy Enqueue Element(queue=w515, element=w513) -> (queue out=w514:refnum<queue>, error out=w512:errorcluster)  [unwired: 1 in, 2 out]
                n196 = Lossy Enqueue Element(queue=w536, element=w534, error in (no error)=w508) -> (error out=w507:errorcluster)  [unwired: 3 out]
                n197 = flat-sequence {
                  tunnel: w530 -> [w548]
                  tunnel: [w547] -> w526
                  tunnel: [w546] -> w525
                  tunnel: [w545] -> w524
                  tunnel: [w544] -> w523
                  tunnel: w521 -> [w539]
                  tunnel: w520 -> [w543]
                  tunnel: 0 -> [w542]
                  tunnel: w507 -> [_]
                  tunnel: w506 -> [w541]
                  frame #0 {
                    w538 = "1" ("Channel")
                    n198 = call-poly <instrlib>:"niScope Fetch (poly).vi"("timeout"=w542, "numSamples"=w548, "channels"="1" ("Channel"), "instrument handle"=w541) -> ("wfm"=w547:i8[][])  [unwired: 1 in, 6 out]
                    n199 = call-poly <instrlib>:"niScope Fetch (poly).vi"("timeout"=w542, "numSamples"=w548, "instrument handle"=w539) -> ("wfm"=w546:i8[][])  [unwired: 2 in, 6 out]
                    n200 = call-poly <instrlib>:"niScope Fetch (poly).vi"("timeout"=w542, "numSamples"=w548, "channels"=w538, "instrument handle"=w539) -> ("wfm"=w545:i8[][])  [unwired: 1 in, 6 out]
                    n201 = call-poly <instrlib>:"niScope Fetch (poly).vi"("timeout"=w542, "numSamples"=w548, "channels"=w538, "instrument handle"=w543) -> ("wfm"=w544:i8[][])  [unwired: 1 in, 6 out]
                  }
                }
                n202 = Lossy Enqueue Element(queue=w514, element=w526, error in (no error)=w512) -> (queue out=w529:refnum<queue>, error out=w511:errorcluster)  [unwired: 2 out]
                n203 = Lossy Enqueue Element(queue=w529, element=w525, error in (no error)=w511) -> (queue out=w528:refnum<queue>, error out=w510:errorcluster)  [unwired: 2 out]
                n204 = Lossy Enqueue Element(queue=w528, element=w524, error in (no error)=w510) -> (queue out=w527:refnum<queue>, error out=w509:errorcluster)  [unwired: 2 out]
                n205 = Lossy Enqueue Element(queue=w527, element=w523, error in (no error)=w509) -> ()  [unwired: 4 out]
                "Read Data index" <- w519
              }
              n206 = And(x=w443, y=w442) -> (x .and. y?=w414:bool)
              n207 = Release Queue(queue=w441, force destroy? (F)=w414) -> ()  [unwired: 1 in, 3 out]
              n208 = Release Queue(queue=w423, force destroy? (F)=w414) -> ()  [unwired: 1 in, 3 out]
              n209 = Release Queue(queue=w415, force destroy? (F)=w414) -> ()  [unwired: 1 in, 3 out]
            }
            frame "1T/5R Deep Mem" {
              # "1T/5R test case/ This works but was a bit slower than case using flip flop gate. Also cam suffer memory overflow if Byte depth too small"
              # "Arm digitizer"
              n210 = Reverse 1D Array(array=w560) -> (reversed array=w557:void[])
              n211 = for {
                tunnel: [w627] -> w561
                tunnel: w557 -> [w626] mode=indexing
                n212 = call <instrlib>:"niScope Initiate Acquisition.vi"("instrument handle"=w626) -> ("error out"=w627:errorcluster)  [unwired: 2 in, 12 out]
              }
              n213 = Array To Cluster(array=w560) -> (cluster=w564:cluster{"[0]":void, "[1]":void, "[2]":void})
              n214 = Index Array(array=w577) -> (element=w576:T11)  [unwired: 1 in]
              n215 = Index Array(array=w577, index=1) -> (element=w572:T11)
              n216 = Index Array(array=w577, index=2) -> (element=w573:T11)
              n217 = Index Array(array=w577, index=3) -> (element=w574:T11)
              n218 = Index Array(array=w577, index=4) -> (element=w575:T11)
              n219 = Unbundle(w564) -> ("[0]"=w563, "[1]"=w559, "[2]"=w558)
              n220 = Obtain Queue(max queue size (-1, unlimited)=5, element data type=cluster{"Fetch:Records Done":i32, bool} {"Fetch:Records Done"=0, TRUE}) -> (queue out=w569:refnum<queue>)  [unwired: 2 in, 3 out]
              n221 = node-c288() -> (w554:T6)  [unwired: 4 in]
              n222 = Obtain Queue(max queue size (-1, unlimited)=25, element data type=i8[][] [] ("Array")) -> (queue out=w571:refnum<queue>)  [unwired: 2 in, 3 out]
              n223 = while {
                tunnel: w569 -> [w702]
                tunnel: [w693] -> w568
                tunnel: w563 -> [w698]
                tunnel: w559 -> [w690]
                tunnel: w558 -> [w697]
                tunnel: w571 -> [w700]
                tunnel: w583 -> [w671]
                tunnel: w582 -> [w696]
                tunnel: [w674] -> w566
                tunnel: w561 -> [w692]
                tunnel: [w681] -> w549
                i -> [w683]
                stop <- w693 stop-if-true
                w686 = 483 items=["Start"=482, "Trigger"=483, "Pretrigger"=477, "Now"=481, "Read Pointer"=388] ("Fetch:Fetch Relative To")
                w673 = 1
                # "This loop reads the data once it is in the queue"
                # "Get and display data"
                n224 = Dequeue Element(queue=w702, timeout in ms (-1)=10000, error in (no error)=w692) -> (element=w701:cluster{"Fetch:Records Done":i32, bool}, error out=w684:errorcluster)  [unwired: 2 out]
                n225 = local write "Read Data index"(w683) -> ()
                n226 = Unbundle(w701) -> ("Fetch:Records Done"=w687:i32)  [unwired: 1 out]
                n227 = property class="niScope"(reference=w698, error in=w684, "Fetch Relative To"=w686, "Fetch Record Number"=w687, "Fetch Number of Records"=w696) -> (reference out=w680:refnum<k15>, error out=w685:errorcluster)
                n228 = property class="niScope"(reference=w690, "Fetch Relative To"=w686, "Fetch Record Number"=w687, "Fetch Number of Records"=w696) -> (reference out=w688:refnum<k15>)  [unwired: 1 in, 1 out]
                n229 = call-poly <instrlib>:"niScope Fetch (poly).vi"("timeout"=w673, "error in"=w685, "numSamples"=w671, "instrument handle"=w680) -> ("error out"=w682:errorcluster, "wfm"=w691:i8[][])  [unwired: 1 in, 5 out]
                n230 = Lossy Enqueue Element(queue=w700, element=w691, error in (no error)=w682) -> (queue out=w678:refnum<queue>, error out=w679:errorcluster)  [unwired: 2 out]
                n231 = call-poly <instrlib>:"niScope Fetch (poly).vi"("timeout"=w673, "numSamples"=w671, "channels"="1", "instrument handle"=w680) -> ("wfm"=w675:i8[][])  [unwired: 1 in, 6 out]
                n232 = Lossy Enqueue Element(queue=w678, element=w675, error in (no error)=w679) -> (queue out=w676:refnum<queue>, error out=w677:errorcluster)  [unwired: 2 out]
                n233 = property class="niScope"(reference=w697, "Fetch Relative To"=w686, "Fetch Record Number"=w687, "Fetch Number of Records"=w696) -> (reference out=w689:refnum<k15>)  [unwired: 1 in, 1 out]
                n234 = stacked-sequence {
                  tunnel: [w717] -> w705
                  tunnel: [w716] -> w704
                  tunnel: [w715] -> w703
                  tunnel: w671 -> [w714]
                  tunnel: w673 -> [w713]
                  tunnel: w689 -> [w712]
                  tunnel: w688 -> [w711]
                  tunnel: [w708] -> w681
                  frame #0 {
                    n235 = call-poly <instrlib>:"niScope Fetch (poly).vi"("timeout"=w713, "numSamples"=w714, "instrument handle"=w711) -> ("wfm"=w717:i8[][])  [unwired: 2 in, 6 out]
                    n236 = call-poly <instrlib>:"niScope Fetch (poly).vi"("timeout"=w713, "numSamples"=w714, "channels"="1" ("Channel"), "instrument handle"=w711) -> ("wfm"=w716:i8[][])  [unwired: 1 in, 6 out]
                    n237 = call-poly <instrlib>:"niScope Fetch (poly).vi"("timeout"=w713, "numSamples"=w714, "channels"="1" ("Channel"), "instrument handle"=w712) -> ("error out"=w708:errorcluster, "wfm"=w715:i8[][])  [unwired: 1 in, 5 out]
                  }
                }
                n238 = Lossy Enqueue Element(queue=w676, element=w705, error in (no error)=w677) -> (queue out=w707:refnum<queue>, error out=w695:errorcluster)  [unwired: 2 out]
                n239 = local read "stop out"() -> (w693:bool)
                n240 = Lossy Enqueue Element(queue=w707, element=w704, error in (no error)=w695) -> (queue out=w706:refnum<queue>, error out=w694:errorcluster)  [unwired: 2 out]
                n241 = Lossy Enqueue Element(queue=w706, element=w703, error in (no error)=w694) -> (queue out=w674:refnum<queue>)  [unwired: 3 out]
              }
              n242 = timed-loop {
                shift-right: [w600] -> _
                shift-left: 0 -> [w608]
                shift-right: [w615] -> _
                shift-left: TRUE -> [w609]
                tunnel: w586 -> [w613]
                tunnel: w569 -> [w604]
                tunnel: [w607] -> w555
                tunnel: [w594] -> w567
                tunnel: w563 -> [w606]
                tunnel: w562 -> [w601]
                tunnel: w561 -> [w611]
                timing: w554 -> [_]
                timing-out: [_] -> w553
                i -> [w593]
                stop <- w607 stop-if-true
                # "This loop performs back and forth scan and records record # at end of run"
                n243 = Bundle(w608, w609) -> (w605:cluster{i32, bool})  [unwired: 1 in]
                n244 = Select(t=T5 6 ("Program (1)"), s=w609, f=T5 7 ("Program (1)")) -> (s? t:f=w612:T5)
                n245 = call <vilib>:"Run Program.flx"("error in (no error)"=w611, "Program (1)"=w612, "Board ID"=w613) -> ("error out"=w603:errorcluster, "Bd ID Out"=w598:T2)  [unwired: 4 out]
                n246 = stacked-sequence {
                  tunnel: w603 -> [w619]
                  tunnel: [w619] -> w602
                  tunnel: [w617] -> w599
                  tunnel: w598 -> [w617]
                  frame #0 {
                    n247 = Wait (ms)(milliseconds to wait=20) -> ()  [unwired: 1 out]
                  }
                }
                n248 = call-poly <vilib>:"Wait for Move Complete.flx"("Poll Interval (20 ms)"=5, "error in (no error)"=w602, "Axis or Vector Space"=w601, "Board ID"=w599) -> ("error out"=w610:errorcluster)  [unwired: 4 in, 3 out]
                n249 = property class="niScope"(reference=w606, error in=w610) -> (error out=w597:errorcluster, "Records Done"=w600:i32)  [unwired: 1 out]
                n250 = local read "stop out"() -> (w607:bool)
                n251 = Lossy Enqueue Element(queue=w604, element=w605, error in (no error)=w597) -> (queue out=w595:refnum<queue>, error out=w592:errorcluster)  [unwired: 2 out]
                n252 = Not(x=w609) -> (.not. x?=w615:bool)
                n253 = Get Queue Status(queue=w595, error in (no error)=w592) -> (queue out=w594:refnum<queue>, # elements in queue=→"Record queue":i32)  [unwired: 1 in, 6 out]
                "Read Loop" <- w593
              }
              n254 = while {
                tunnel: w571 -> [w667]
                tunnel: [w631] -> w570
                tunnel: w575 -> [w660]
                tunnel: w574 -> [w659]
                tunnel: w576 -> [w658]
                tunnel: w572 -> [w657]
                tunnel: w573 -> [w656]
                tunnel: w561 -> [w646]
                shift-right: [w632] -> _
                shift-left: TRUE -> [w630]
                tunnel: w551 -> [w633]
                tunnel: u16 13 ("bits A/D") -> [w629]
                i -> [w635]
                stop <- w631 stop-if-true
                w641 = 100
                # "This loop does beam forming after data is read."
                n255 = Dequeue Element(queue=w667, timeout in ms (-1)=10000, error in (no error)=w646) -> (queue out=w647:refnum<queue>, element=w648:i8[][], error out=w650:errorcluster)  [unwired: 1 out]
                n256 = Dequeue Element(queue=w647, timeout in ms (-1)=w641, error in (no error)=w650) -> (queue out=w666:refnum<queue>, element=w663:i8[][], error out=w645:errorcluster)  [unwired: 1 out]
                n257 = call "TimeShiftData.vi"("output cluster"=w657, "Array In"=w663) -> ("Array Out"=w654:i16[][])  [unwired: 2 in]
                n258 = call "TimeShiftData.vi"("output cluster"=w658, "Array In"=w648) -> ("Array Out"=w655:i16[][])  [unwired: 2 in]
                n259 = Dequeue Element(queue=w666, timeout in ms (-1)=w641, error in (no error)=w645) -> (queue out=w665:refnum<queue>, element=w662:i8[][], error out=w644:errorcluster)  [unwired: 1 out]
                n260 = call "TimeShiftData.vi"("output cluster"=w656, "Array In"=w662) -> ("Array Out"=w653:i16[][])  [unwired: 2 in]
                n261 = Dequeue Element(queue=w665, timeout in ms (-1)=w641, error in (no error)=w644) -> (queue out=w664:refnum<queue>, element=w643:i8[][], error out=w642:errorcluster)  [unwired: 1 out]
                n262 = call "TimeShiftData.vi"("output cluster"=w659, "Array In"=w643) -> ("Array Out"=w652:i16[][])  [unwired: 2 in]
                n263 = Dequeue Element(queue=w664, timeout in ms (-1)=w641, error in (no error)=w642) -> (queue out=w640:refnum<queue>, element=w661:i8[][], error out=w639:errorcluster)  [unwired: 1 out]
                n264 = call "TimeShiftData.vi"("output cluster"=w660, "Array In"=w661) -> ("Array Out"=w651:i16[][])  [unwired: 2 in]
                n265 = Get Queue Status(queue=w640, error in (no error)=w639) -> (# elements in queue=→"SF queue":i32)  [unwired: 1 in, 7 out]
                n266 = Compound Arithmetic op=ADD(w655, w654, w653, w652, w651) -> (w634:i16[][])
                n267 = case shown="True" w630 {
                  tunnel: [w668 w670] -> w636
                  tunnel: w634 -> [w668 w669]
                  frame False {
                  }
                  frame True {
                    n268 = call "ReverseData.vi"("Array in"=w669) -> ("Array out"=w670:i16[][])
                  }
                }
                n269 = Increment(x=w635) -> (x+1=w637:i32)
                n270 = local write "SF Index"(w635) -> ()
                n271 = call "CurrentPlane.vi"("gain"=1.0, "bits A/D"=w629, "Axis Vals"=w633, "Frame"=w637, "Data"=w636) -> ("stop out"=w631:bool)  [unwired: 5 in, 1 out]
                n272 = local write "stop out"(w631) -> ()
                n273 = Not(x=w630) -> (.not. x?=w632:bool)
              }
              n274 = node-c288(w553) -> ()
              n275 = Compound Arithmetic op=AND(w555, w568, w570) -> (w556:bool)
              n276 = Release Queue(queue=w567, force destroy? (F)=w556) -> ()  [unwired: 1 in, 3 out]
              n277 = for {
                tunnel: w560 -> [w625]
                tunnel: w549 -> [w624]
                n278 = call <instrlib>:"niScope Abort.vi"("instrument handle"=w625, "error in"=w624) -> ()  [unwired: 12 in, 2 out]
              }
              n279 = Release Queue(queue=w566, force destroy? (F)=w556) -> ()  [unwired: 1 in, 3 out]
            }
            frame "Full 25 Ch" {
              w734 = 10
              w729 = 2 ("index")
              w757 = 5
              w736 = "0,1"
              # "Restructure file names"
              # "Read queue and send to files. About same as reading channel by channel"
              n280 = Reshape Array(w758, w757, w757) -> (w727:T12)
              n281 = expression code="x*5"(w748) -> (w759:dbl)
              n282 = Index Array(array=w720, index=2) -> (element=w718)
              n283 = Index Array(array=w727, index (col)=4 ("index")) -> (element=w733:T13)  [unwired: 1 in]
              n284 = Initialize Array(i16 0, w748, w726) -> (w746:i16[][])
              n285 = Index Array(array=w720, index=1) -> (element=w719)
              n286 = Array Subset(array=w727, index (col)=w729, length (col)=w729) -> (w732:T12)  [unwired: 2 in]
              n287 = Array Subset(array=w727, length (col)=2 ("index")) -> (w731:T12)  [unwired: 3 in]
              n288 = call "RTHeader.vi"("Comment"="Full 25") -> ("Header String Out"=w723:string)  [unwired: 5 in, 1 out]
              n289 = Obtain Queue(max queue size (-1, unlimited)=3, element data type=T9 {"gain"=0.0, "wfm"=[], TRUE, "max queue size (-1, unlimited)"=15}) -> (queue out=w761:refnum<queue>)  [unwired: 3 in, 2 out]
              n290 = New Data Value Reference(data value=w746) -> (data value reference=w745:refnum<data-value>)  [unwired: 1 in, 1 out]
              n291 = Reshape Array(w731, w734) -> (w735:T13)
              n292 = Reshape Array(w732, w734) -> (w743:T13)
              n293 = Obtain Queue(max queue size (-1, unlimited)=3, element data type=cluster{"gain":dbl, bool, "wfm":i16[][]} {"gain"=0.0, TRUE, "wfm"=[]}) -> (queue out=w747:refnum<queue>)  [unwired: 3 in, 2 out]
              n294 = Build Array(w736, w736, "1") -> (w763:string[])
              n295 = Tick Count (ms)() -> (millisecond timer value=w740:u32)
              n296 = Build Array(w735, w743, w733) -> (w742:T12)
              n297 = while {
                tunnel: w761 -> [w782]
                tunnel: w726 -> [w781]
                tunnel: [w777] -> w752
                tunnel: w748 -> [w780]
                tunnel: w745 -> [w776]
                tunnel: w747 -> [w779]
                tunnel: w742 -> [w771]
                tunnel: i32[] [10, 10, 5] -> [w775]
                shift-right: [w773] -> _
                shift-left: w740 -> [w774]
                tunnel: [w772] -> _
                tunnel: 10000 -> [w767]
                tunnel: [w766] -> w725
                tunnel: w723 -> [w764]
                i -> [w765]
                stop <- w777 stop-if-true
                n298 = for {
                  tunnel: w781 -> [w796]
                  tunnel: w780 -> [w806]
                  tunnel: w782 -> [w809]
                  tunnel: [w805] -> w770 mode=indexing
                  tunnel: [w795] -> w778
                  tunnel: [w804] -> w768
                  tunnel: w776 -> [w803]
                  tunnel: w771 -> [_] mode=indexing
                  tunnel: w775 -> [w799]
                  tunnel: w771 -> [w801]
                  tunnel: w767 -> [w798]
                  tunnel: w765 -> [w793]
                  tunnel: w764 -> [w791]
                  n299 = Dequeue Element(queue=w809, timeout in ms (-1)=w798) -> (element=w808:T9)  [unwired: 1 in, 3 out]
                  n300 = Unbundle(w808) -> ("gain"=w795:dbl, "wfm"=w792:i8[][], w805:bool, "max queue size (-1, unlimited)"=w790:i32)
                  n301 = Index Array(array=w799, index=w790) -> (element=w797:i32)
                  n302 = Index Array(array=w801, index (row)=w790) -> (element=w800:T13)  [unwired: 1 in]
                  n303 = Multiply(x=w796, y=w797) -> (x*y=w802:i32)
                  n304 = Reshape Array(w792, w806, w802) -> (w807:i8[][])
                  n305 = for {
                    N: w797 -> [_]
                    tunnel: w800 -> [w821]
                    tunnel: [w824] -> w804
                    tunnel: w803 -> [w823]
                    shift-right: [w816] -> _
                    shift-left: w807 -> [w826]
                    tunnel: w796 -> [w815]
                    i -> [w822]
                    n306 = Index Array(array=w821, index=w822) -> (element=w820:T11)
                    n307 = Delete From Array(array=w826, length=w815, index (col)=0 ("disabled index (col)")) -> (deleted portion=w819:i8[], array with subset deleted=w816:i8[][])  [unwired: 1 in]
                    n308 = for {
                      tunnel: w819 -> [w828] mode=indexing
                      tunnel: [w827] -> w818 mode=indexing
                      n309 = call-poly <vilib>:"Mean.vi"("X"=w828) -> ("mean"=w830:dbl)  [unwired: 1 out]
                      n310 = To Word Integer(number=w830) -> (16bit integer=w829:i16)
                      n311 = Subtract(x=w828, y=w829) -> (x-y=w827:i16)
                    }
                    n312 = call-poly "TimeShiftDataPoly.vi"("output cluster"=w820, "Array In"=w818) -> ("Array Out"=w825:i16[][])  [unwired: 2 in]
                    n313 = in-place {
                      in-place-border: w825 -> [w833]
                      n314 = in-place-dvr #1(w823) -> (w831:i16[][])  [unwired: 1 out]
                      n315 = Add(x=w833, y=w831) -> (x+y=w832:i16[][])
                      n316 = in-place-dvr #1(w832) -> (w824:refnum<data-value>)  [unwired: 1 out]
                    }
                  }
                  n317 = case shown="True" "Save Raw" {
                    tunnel: w790 -> [_ w811]
                    tunnel: w793 -> [_ w813]
                    tunnel: w792 -> [_ w810]
                    tunnel: w791 -> [_ w812]
                    frame False {
                    }
                    frame True {
                      n318 = call "RawRT_Capture.vi"("Raw data"=w810, "File Name In"="Raw Name", "DigCard"=w811, "header"=w812, "Iter"=w813) -> ()  [unwired: 7 in]
                    }
                  }
                }
                n319 = local write "SF Index"(w765) -> ()
                n320 = local read "stop out"() -> (w777:bool)
                n321 = Or Array Elements(Boolean array=w770) -> (logical OR=w769:bool)
                n322 = in-place {
                  in-place-border: w779 -> [w789]
                  in-place-border: w769 -> [w788]
                  in-place-border: w778 -> [w787]
                  n323 = in-place-dvr #2(w768) -> (w783:i16[][])  [unwired: 1 out]
                  n324 = Bundle("gain"=w787, w788, w783) -> (w786:cluster{"gain":dbl, bool, i16[][]})  [unwired: 1 in]
                  n325 = Multiply(x=i16 0, y=w783) -> (x*y=w785:i16[][])
                  n326 = Enqueue Element(queue=w789, element=w786) -> ()  [unwired: 2 in, 3 out]
                  n327 = in-place-dvr #2(w785) -> (w766:refnum<data-value>)  [unwired: 1 out]
                }
                n328 = Tick Count (ms)() -> (millisecond timer value=w773:u32)
                n329 = Subtract(x=w773, y=w774) -> (x-y=w772:u32)
              }
              n330 = while {
                tunnel: w750 -> [w900]
                tunnel: w747 -> [w894]
                tunnel: [w897] -> _
                tunnel: [w899] -> w751
                i -> [w901]
                stop <- w897 stop-if-true
                # "Slightly faster version to read data"
                # "Get and display data"
                n331 = Dequeue Element(queue=w894, timeout in ms (-1)=5000) -> (queue out=w899:refnum<queue>, element=w896:cluster{"gain":dbl, bool, "wfm":i16[][]})  [unwired: 1 in, 2 out]
                n332 = Unbundle(w896) -> ("gain"=w891:dbl, w892:bool, "wfm"=w893:i16[][])
                n333 = case shown="True" w892 {
                  tunnel: w893 -> [w902 w904]
                  tunnel: [w902 w903] -> w895
                  frame False {
                  }
                  frame True {
                    n334 = call "ReverseData.vi"("Array in"=w904) -> ("Array out"=w903:i16[][])
                  }
                }
                n335 = Increment(x=w901) -> (x+1=w890:i32)
                n336 = local write "Display index"(w890) -> ()
                n337 = call "CurrentPlane.vi"("gain"=w891, "bits A/D"=13, "Axis Vals"=w900, "Frame"=w890, "Data"=w895) -> ("stop out"=w897:bool)  [unwired: 5 in, 1 out]
                n338 = local write "stop out"(w897) -> ()
              }
              n339 = global read "MotionGlobals.vi" "DigTimeOut"() -> (w739)
              n340 = while {
                tunnel: w720 -> [w847]
                tunnel: w763 -> [w846]
                tunnel: w761 -> [w845]
                tunnel: w719 -> [w844]
                tunnel: w718 -> [w843]
                tunnel: w759 -> [w842]
                tunnel: w726 -> [w841]
                tunnel: [w840] -> w753
                tunnel: w744 -> [w838]
                shift-right: [w836] -> _
                shift-left: w740 -> [w837]
                tunnel: [w835] -> _
                tunnel: w739 -> [w834]
                stop <- w839 stop-if-true
                n341 = for {
                  tunnel: w841 -> [w860]
                  tunnel: w842 -> [w863]
                  tunnel: w847 -> [w862]
                  tunnel: w846 -> [w861] mode=indexing
                  tunnel: w845 -> [w859]
                  tunnel: [w855] -> _
                  tunnel: w844 -> [w854]
                  tunnel: w843 -> [w853]
                  tunnel: [w851] -> w840
                  tunnel: w838 -> [w850]
                  tunnel: w834 -> [w849]
                  i -> [w848]
                  # "Read data"
                  n342 = case shown="0" w848 {
                    tunnel: w863 -> [_ w885]
                    tunnel: w862 -> [w867 w884]
                    tunnel: w861 -> [w865 w882]
                    tunnel: w860 -> [w868 w881]
                    tunnel: [w869 w880] -> w858
                    tunnel: [w871 w879] -> w857
                    tunnel: [w870 w878] -> w855
                    tunnel: w854 -> [w875 _]
                    tunnel: w853 -> [w874 _]
                    tunnel: [w866 _] -> w852
                    tunnel: w850 -> [w864 _]
                    tunnel: w849 -> [_ w876]
                    frame 0 {
                      # "Read files and queue it up."
                      n343 = call <instrlib>:"niScope Initiate Acquisition.vi"("instrument handle"=w875) -> ("error out"=w873:errorcluster)  [unwired: 2 in, 12 out]
                      n344 = call <instrlib>:"niScope Initiate Acquisition.vi"("instrument handle"=w874, "error in"=w873) -> ("error out"=w872:errorcluster)  [unwired: 1 in, 12 out]
                      n345 = call "Rapid Read_NI.vi"("NI Card"=w867, "Channel"=w865, "Motion Board ID"=w864, "rf points per line"=w868, "error in"=w872) -> ("dig gain"=w869:dbl, "Array"=w871:i8[][], "Reverse?"=w866:bool, "error out"=w870:errorcluster)  [unwired: 7 in]
                    }
                    frame 1, Default {
                      n346 = property class="niScope"(reference=w884, "Fetch Record Number"=0, "Fetch Number of Records"=w885) -> (reference out=w883:refnum<k15>, error out=w877:errorcluster)  [unwired: 1 in]
                      n347 = call-poly <instrlib>:"niScope Fetch (poly).vi"("timeout"=w876, "error in"=w877, "numSamples"=w881, "channels"=w882, "instrument handle"=w883) -> ("error out"=w878:errorcluster, "wfm"=w879:i8[][], "wfm info"=w888:T14)  [unwired: 4 out]
                      n348 = Index Array(array=w888) -> (element=w887:T15)  [unwired: 1 in]
                      n349 = Unbundle By Name(w887) -> ("gain"=w880:dbl)
                    }
                  }
                  n350 = local write "Read Data index"(w848) -> ()
                  n351 = Bundle("gain"=w858, "wfm"=w857, "Reverse?"=w852, w848) -> (w856:T16)  [unwired: 1 in]
                  n352 = Enqueue Element(queue=w859, element=w856) -> (queue out=w851:refnum<queue>)  [unwired: 2 in, 2 out]
                }
                n353 = local read "stop out"() -> (w839:bool)
                n354 = Tick Count (ms)() -> (millisecond timer value=w836:u32)
                n355 = Subtract(x=w836, y=w837) -> (x-y=w835:u32)
              }
              n356 = Release Queue(queue=w753, force destroy? (F)=w752) -> ()  [unwired: 1 in, 3 out]
              n357 = Delete Data Value Reference(data value reference=w725) -> ()  [unwired: 1 in, 2 out]
              n358 = Release Queue(queue=w751, force destroy? (F)=w752) -> ()  [unwired: 1 in, 3 out]
            }
            frame "Drop Ch 5" {
              w917 = 2 ("index")
              w942 = 5
              # "Reduced data case that drop ring 5 receive"
              # "Restructure file names"
              # "Read queue and send to files. About same as reading channel by channel"
              n359 = Reshape Array(w943, w942, w942) -> (w915:T12)
              n360 = Index Array(array=w906, index=1) -> (element=w905)
              n361 = Array Subset(array=w906, length=2) -> (w908:void[])  [unwired: 1 in]
              n362 = Initialize Array(i16 0, w912, w914) -> (w932:i16[][])
              n363 = Array Subset(array=w915, index (col)=w917, length (col)=w917) -> (w916:T12)  [unwired: 2 in]
              n364 = Array Subset(array=w915, length (col)=2 ("index")) -> (w919:T12)  [unwired: 3 in]
              n365 = Obtain Queue(max queue size (-1, unlimited)=3, element data type=T9 {"gain"=0.0, "wfm"=[], TRUE, "max queue size (-1, unlimited)"=15}) -> (queue out=w945:refnum<queue>)  [unwired: 3 in, 2 out]
              n366 = New Data Value Reference(data value=w932) -> (data value reference=w931:refnum<data-value>)  [unwired: 1 in, 1 out]
              n367 = Reshape Array(w919, 10) -> (w918:T13)
              n368 = Reshape Array(w916, 10) -> (w929:T13)
              n369 = Obtain Queue(max queue size (-1, unlimited)=3, element data type=cluster{"gain":dbl, bool, "wfm":i16[][]} {"gain"=0.0, TRUE, "wfm"=[]}) -> (queue out=w933:refnum<queue>)  [unwired: 3 in, 2 out]
              n370 = expression code="x*5"(w912) -> (w910:dbl)
              n371 = Tick Count (ms)() -> (millisecond timer value=w926:u32)
              n372 = Build Array(w918, w929) -> (w928:T12)
              n373 = while {
                tunnel: w945 -> [w965]
                tunnel: w914 -> [w964]
                tunnel: [w960] -> w937
                tunnel: w912 -> [w963]
                tunnel: w931 -> [w958]
                tunnel: w933 -> [w962]
                tunnel: w928 -> [w953]
                tunnel: i32[] [10, 10] -> [w957]
                shift-right: [w955] -> _
                shift-left: w926 -> [w956]
                tunnel: [w954] -> _
                tunnel: 10000 -> [w949]
                tunnel: i16[] [1, 1, 1, 1, 1, 1, 1, 1, 2, 2] -> [w948]
                tunnel: [w947] -> w913
                i -> [w959]
                stop <- w960 stop-if-true
                n374 = for {
                  tunnel: w964 -> [w976]
                  tunnel: w963 -> [w987]
                  tunnel: w965 -> [w990]
                  tunnel: [w986] -> w952 mode=indexing
                  tunnel: [w985] -> w961
                  tunnel: [w984] -> w950
                  tunnel: w958 -> [w983]
                  tunnel: w953 -> [_] mode=indexing
                  tunnel: w957 -> [w980]
                  tunnel: w953 -> [w982]
                  tunnel: w949 -> [w979]
                  tunnel: w948 -> [w975]
                  n375 = Dequeue Element(queue=w990, timeout in ms (-1)=w979) -> (element=w989:T9)  [unwired: 1 in, 3 out]
                  n376 = Unbundle(w989) -> ("gain"=w985:dbl, "wfm"=w988:i8[][], w986:bool, "max queue size (-1, unlimited)"=w977:i32)
                  n377 = Index Array(array=w980, index=w977) -> (element=w978:i32)
                  n378 = Index Array(array=w982, index (row)=w977) -> (element=w981:T13)  [unwired: 1 in]
                  n379 = Multiply(x=w976, y=w978) -> (x*y=w974:i32)
                  n380 = Reshape Array(w988, w987, w974) -> (w973:i8[][])
                  n381 = for {
                    N: w978 -> [_]
                    tunnel: w981 -> [w998]
                    tunnel: [w1001] -> w984
                    tunnel: w983 -> [w1000]
                    shift-right: [w991] -> _
                    shift-left: w973 -> [w1003]
                    tunnel: w975 -> [w993] mode=indexing
                    tunnel: w976 -> [w992]
                    i -> [w999]
                    n382 = Index Array(array=w998, index=w999) -> (element=w997:T11)
                    n383 = Delete From Array(array=w1003, length=w992, index (col)=0 ("disabled index (col)")) -> (deleted portion=w996:i8[], array with subset deleted=w991:i8[][])  [unwired: 1 in]
                    n384 = for {
                      tunnel: w996 -> [w1006] mode=indexing
                      tunnel: [w1005] -> w995 mode=indexing
                      n385 = call-poly <vilib>:"Mean.vi"("X"=w1006) -> ("mean"=w1007:dbl)  [unwired: 1 out]
                      n386 = To Word Integer(number=w1007) -> (16bit integer=w1004:i16)
                      n387 = Subtract(x=w1006, y=w1004) -> (x-y=w1005:i16)
                    }
                    n388 = call-poly "TimeShiftDataPoly.vi"("output cluster"=w997, "Array In"=w995) -> ("Array Out"=w1002:i16[][])  [unwired: 2 in]
                    n389 = in-place {
                      in-place-border: w1002 -> [w1009]
                      in-place-border: w993 -> [w1010]
                      n390 = in-place-dvr #3(w1000) -> (w1011:i16[][])  [unwired: 1 out]
                      n391 = case shown="2" w1010 {
                        selector: w1010 -> [_ w1014]
                        tunnel: w1009 -> [w1013 w1016]
                        tunnel: [w1013 w1015] -> w1008
                        frame 0, Default {
                        }
                        frame 2 {
                          n392 = Multiply(x=w1014, y=w1016) -> (x*y=w1015:i16[][])
                        }
                      }
                      n393 = Add(x=w1008, y=w1011) -> (x+y=w1012:i16[][])
                      n394 = in-place-dvr #3(w1012) -> (w1001:refnum<data-value>)  [unwired: 1 out]
                    }
                  }
                }
                n395 = local write "SF Index"(w959) -> ()
                n396 = local read "stop out"() -> (w960:bool)
                n397 = Or Array Elements(Boolean array=w952) -> (logical OR=w951:bool)
                n398 = in-place {
                  in-place-border: w962 -> [w972]
                  in-place-border: w951 -> [w971]
                  in-place-border: w961 -> [w970]
                  n399 = in-place-dvr #4(w950) -> (w966:i16[][])  [unwired: 1 out]
                  n400 = Bundle("gain"=w970, w971, w966) -> (w969:cluster{"gain":dbl, bool, i16[][]})  [unwired: 1 in]
                  n401 = Multiply(x=i16 0, y=w966) -> (x*y=w968:i16[][])
                  n402 = Enqueue Element(queue=w972, element=w969) -> ()  [unwired: 2 in, 3 out]
                  n403 = in-place-dvr #4(w968) -> (w947:refnum<data-value>)  [unwired: 1 out]
                }
                n404 = Tick Count (ms)() -> (millisecond timer value=w955:u32)
                n405 = Subtract(x=w955, y=w956) -> (x-y=w954:u32)
              }
              n406 = while {
                tunnel: w935 -> [w1079]
                tunnel: w933 -> [w1073]
                tunnel: [w1076] -> _
                tunnel: [w1078] -> w936
                i -> [w1080]
                stop <- w1076 stop-if-true
                # "Slightly faster version to read data"
                # "Get and display data"
                n407 = Dequeue Element(queue=w1073, timeout in ms (-1)=5000) -> (queue out=w1078:refnum<queue>, element=w1075:cluster{"gain":dbl, bool, "wfm":i16[][]})  [unwired: 1 in, 2 out]
                n408 = Unbundle(w1075) -> ("gain"=w1070:dbl, w1071:bool, "wfm"=w1072:i16[][])
                n409 = case shown="False" w1071 {
                  tunnel: w1072 -> [w1081 w1083]
                  tunnel: [w1081 w1082] -> w1074
                  frame False {
                  }
                  frame True {
                    n410 = call "ReverseData.vi"("Array in"=w1083) -> ("Array out"=w1082:i16[][])
                  }
                }
                n411 = Increment(x=w1080) -> (x+1=w1069:i32)
                n412 = local write "Display index"(w1069) -> ()
                n413 = call "CurrentPlane.vi"("gain"=w1070, "bits A/D"=13, "Axis Vals"=w1079, "Frame"=w1069, "Data"=w1074) -> ("stop out"=w1076:bool)  [unwired: 5 in, 1 out]
                n414 = local write "stop out"(w1076) -> ()
              }
              n415 = global read "MotionGlobals.vi" "DigTimeOut"() -> (w925)
              n416 = while {
                tunnel: w908 -> [w1029]
                tunnel: w945 -> [w1028]
                tunnel: w905 -> [w1027]
                tunnel: w914 -> [w1026]
                tunnel: [w1025] -> w938
                tunnel: w930 -> [w1023]
                shift-right: [w1021] -> _
                shift-left: w926 -> [w1022]
                tunnel: [w1020] -> _
                tunnel: w925 -> [w1019]
                tunnel: "0,1" -> [w1018]
                tunnel: w910 -> [w1017]
                stop <- w1024 stop-if-true
                n417 = for {
                  tunnel: w1026 -> [w1042]
                  tunnel: w1029 -> [w1044] mode=indexing
                  tunnel: w1018 -> [w1043]
                  tunnel: w1028 -> [w1041]
                  tunnel: [w1037] -> _
                  tunnel: w1027 -> [w1036]
                  tunnel: [w1034] -> w1025
                  tunnel: w1023 -> [w1033]
                  tunnel: w1019 -> [w1032]
                  tunnel: w1017 -> [w1030]
                  i -> [w1031]
                  # "Read data"
                  n418 = case shown="0" w1031 {
                    tunnel: w1044 -> [w1050 w1059]
                    tunnel: w1043 -> [w1048 w1058]
                    tunnel: w1042 -> [w1051 w1064]
                    tunnel: [w1052 w1063] -> w1040
                    tunnel: [w1045 w1057] -> w1039
                    tunnel: [w1053 w1062] -> w1037
                    tunnel: w1036 -> [w1054 _]
                    tunnel: [w1049 _] -> w1035
                    tunnel: w1033 -> [w1047 _]
                    tunnel: w1032 -> [_ w1060]
                    tunnel: w1030 -> [_ w1055]
                    frame 0 {
                      # "Read files and queue it up."
                      n419 = call <instrlib>:"niScope Initiate Acquisition.vi"("instrument handle"=w1054) -> ("error out"=w1046:errorcluster)  [unwired: 2 in, 12 out]
                      n420 = call "Rapid Read_NI.vi"("NI Card"=w1050, "Channel"=w1048, "Motion Board ID"=w1047, "rf points per line"=w1051, "error in"=w1046) -> ("dig gain"=w1052:dbl, "Array"=w1045:i8[][], "Reverse?"=w1049:bool, "error out"=w1053:errorcluster)  [unwired: 7 in]
                    }
                    frame 1, Default {
                      n421 = property class="niScope"(reference=w1059, "Fetch Record Number"=0, "Fetch Number of Records"=w1055) -> (reference out=w1065:refnum<k15>, error out=w1061:errorcluster)  [unwired: 1 in]
                      n422 = call-poly <instrlib>:"niScope Fetch (poly).vi"("timeout"=w1060, "error in"=w1061, "numSamples"=w1064, "channels"=w1058, "instrument handle"=w1065) -> ("error out"=w1062:errorcluster, "wfm"=w1057:i8[][], "wfm info"=w1067:T14)  [unwired: 4 out]
                      n423 = Index Array(array=w1067) -> (element=w1066:T15)  [unwired: 1 in]
                      n424 = Unbundle By Name(w1066) -> ("gain"=w1063:dbl)
                    }
                  }
                  n425 = local write "Read Data index"(w1031) -> ()
                  n426 = Bundle("gain"=w1040, "wfm"=w1039, "Reverse?"=w1035, w1031) -> (w1038:T16)  [unwired: 1 in]
                  n427 = Enqueue Element(queue=w1041, element=w1038) -> (queue out=w1034:refnum<queue>)  [unwired: 2 in, 2 out]
                }
                n428 = local read "stop out"() -> (w1024:bool)
                n429 = Tick Count (ms)() -> (millisecond timer value=w1021:u32)
                n430 = Subtract(x=w1021, y=w1022) -> (x-y=w1020:u32)
              }
              n431 = Release Queue(queue=w938, force destroy? (F)=w937) -> ()  [unwired: 1 in, 3 out]
              n432 = Release Queue(queue=w936, force destroy? (F)=w937) -> ()  [unwired: 1 in, 3 out]
              n433 = Delete Data Value Reference(data value reference=w913) -> ()  [unwired: 1 in, 2 out]
            }
            frame "Drop Ch 5,4" {
              w1123 = 5
              # "Reduced data case that drop ring 4,5 receive"
              # "Restructure file names"
              # "Read queue and send to files. About same as reading channel by channel"
              n434 = Reshape Array(w1124, w1123, w1123) -> (w1096:T12)
              n435 = Index Array(array=w1084, index=1) -> (element=w1085)
              n436 = Array Subset(array=w1084, length=2) -> (w1086:void[])  [unwired: 1 in]
              n437 = Initialize Array(i16 0, w1093, w1095) -> (w1113:i16[][])
              n438 = Array Subset(array=w1096, index (col)=2 ("index"), length (col)=1 ("index")) -> (w1097:T12)  [unwired: 2 in]
              n439 = Array Subset(array=w1096, length (col)=2 ("index")) -> (w1100:T12)  [unwired: 3 in]
              n440 = Obtain Queue(max queue size (-1, unlimited)=3, element data type=T9 {"gain"=0.0, "wfm"=[], TRUE, "max queue size (-1, unlimited)"=15}) -> (queue out=w1126:refnum<queue>)  [unwired: 3 in, 2 out]
              n441 = New Data Value Reference(data value=w1113) -> (data value reference=w1112:refnum<data-value>)  [unwired: 1 in, 1 out]
              n442 = Reshape Array(w1100, 10) -> (w1099:T13)
              n443 = Reshape Array(w1097, 5) -> (w1110:T13)
              n444 = Obtain Queue(max queue size (-1, unlimited)=3, element data type=cluster{"gain":dbl, bool, "wfm":i16[][]} {"gain"=0.0, TRUE, "wfm"=[]}) -> (queue out=w1114:refnum<queue>)  [unwired: 3 in, 2 out]
              n445 = expression code="x*5"(w1093) -> (w1092:dbl)
              n446 = Tick Count (ms)() -> (millisecond timer value=w1107:u32)
              n447 = Build Array(w1099, w1110) -> (w1109:T12)
              n448 = while {
                tunnel: w1126 -> [w1147]
                tunnel: w1095 -> [w1146]
                tunnel: [w1142] -> w1118
                tunnel: w1093 -> [w1145]
                tunnel: w1112 -> [w1140]
                tunnel: w1114 -> [w1144]
                tunnel: w1109 -> [w1135]
                tunnel: i32[] [10, 5] -> [w1139]
                shift-right: [w1137] -> _
                shift-left: w1107 -> [w1138]
                tunnel: [w1136] -> _
                tunnel: 10000 -> [w1131]
                tunnel: i16[] [1, 1, 1, 1, 1, 1, 2, 2, 2, 2] -> [w1130]
                tunnel: [w1129] -> w1094
                tunnel: i16[] [1, 1, 1, 2, 2] -> [w1128]
                i -> [w1141]
                stop <- w1142 stop-if-true
                n449 = for {
                  tunnel: w1146 -> [w1161]
                  tunnel: w1145 -> [w1171]
                  tunnel: w1147 -> [w1174]
                  tunnel: [w1170] -> w1134 mode=indexing
                  tunnel: [w1169] -> w1143
                  tunnel: [w1168] -> w1132
                  tunnel: w1140 -> [w1167]
                  tunnel: w1135 -> [_] mode=indexing
                  tunnel: w1139 -> [w1164]
                  tunnel: w1135 -> [w1166]
                  tunnel: w1131 -> [w1163]
                  tunnel: w1130 -> [w1156]
                  tunnel: w1128 -> [w1155]
                  n450 = Dequeue Element(queue=w1174, timeout in ms (-1)=w1163) -> (element=w1173:T9)  [unwired: 1 in, 3 out]
                  n451 = Unbundle(w1173) -> ("gain"=w1169:dbl, "wfm"=w1172:i8[][], w1170:bool, "max queue size (-1, unlimited)"=w1158:i32)
                  n452 = Index Array(array=w1164, index=w1158) -> (element=w1162:i32)
                  n453 = Index Array(array=w1166, index (row)=w1158) -> (element=w1165:T13)  [unwired: 1 in]
                  n454 = case shown="1" w1158 {
                    tunnel: [w1175 w1176] -> w1157
                    tunnel: w1156 -> [w1175 _]
                    tunnel: w1155 -> [_ w1176]
                    frame 0, Default {
                    }
                    frame 1 {
                    }
                  }
                  n455 = Multiply(x=w1161, y=w1162) -> (x*y=w1160:i32)
                  n456 = Reshape Array(w1172, w1171, w1160) -> (w1159:i8[][])
                  n457 = for {
                    N: w1162 -> [_]
                    tunnel: w1165 -> [w1184]
                    tunnel: [w1187] -> w1168
                    tunnel: w1167 -> [w1186]
                    shift-right: [w1177] -> _
                    shift-left: w1159 -> [w1189]
                    tunnel: w1157 -> [w1179] mode=indexing
                    tunnel: w1161 -> [w1178]
                    i -> [w1185]
                    n458 = Index Array(array=w1184, index=w1185) -> (element=w1183:T11)
                    n459 = Delete From Array(array=w1189, length=w1178, index (col)=0 ("disabled index (col)")) -> (deleted portion=w1182:i8[], array with subset deleted=w1177:i8[][])  [unwired: 1 in]
                    n460 = for {
                      tunnel: w1182 -> [w1192] mode=indexing
                      tunnel: [w1191] -> w1181 mode=indexing
                      n461 = call-poly <vilib>:"Mean.vi"("X"=w1192) -> ("mean"=w1193:dbl)  [unwired: 1 out]
                      n462 = To Word Integer(number=w1193) -> (16bit integer=w1190:i16)
                      n463 = Subtract(x=w1192, y=w1190) -> (x-y=w1191:i16)
                    }
                    n464 = call-poly "TimeShiftDataPoly.vi"("output cluster"=w1183, "Array In"=w1181) -> ("Array Out"=w1188:i16[][])  [unwired: 2 in]
                    n465 = in-place {
                      in-place-border: w1188 -> [w1195]
                      in-place-border: w1179 -> [w1196]
                      n466 = in-place-dvr #5(w1186) -> (w1197:i16[][])  [unwired: 1 out]
                      n467 = case shown="2" w1196 {
                        selector: w1196 -> [_ w1200]
                        tunnel: w1195 -> [w1199 w1202]
                        tunnel: [w1199 w1201] -> w1194
                        frame 0, Default {
                        }
                        frame 2 {
                          n468 = Multiply(x=w1200, y=w1202) -> (x*y=w1201:i16[][])
                        }
                      }
                      n469 = Add(x=w1194, y=w1197) -> (x+y=w1198:i16[][])
                      n470 = in-place-dvr #5(w1198) -> (w1187:refnum<data-value>)  [unwired: 1 out]
                    }
                  }
                }
                n471 = local write "SF Index"(w1141) -> ()
                n472 = local read "stop out"() -> (w1142:bool)
                n473 = Or Array Elements(Boolean array=w1134) -> (logical OR=w1133:bool)
                n474 = in-place {
                  in-place-border: w1144 -> [w1154]
                  in-place-border: w1133 -> [w1153]
                  in-place-border: w1143 -> [w1152]
                  n475 = in-place-dvr #6(w1132) -> (w1148:i16[][])  [unwired: 1 out]
                  n476 = Bundle("gain"=w1152, w1153, w1148) -> (w1151:cluster{"gain":dbl, bool, i16[][]})  [unwired: 1 in]
                  n477 = Multiply(x=i16 0, y=w1148) -> (x*y=w1150:i16[][])
                  n478 = Enqueue Element(queue=w1154, element=w1151) -> ()  [unwired: 2 in, 3 out]
                  n479 = in-place-dvr #6(w1150) -> (w1129:refnum<data-value>)  [unwired: 1 out]
                }
                n480 = Tick Count (ms)() -> (millisecond timer value=w1137:u32)
                n481 = Subtract(x=w1137, y=w1138) -> (x-y=w1136:u32)
              }
              n482 = while {
                tunnel: w1116 -> [w1265]
                tunnel: w1114 -> [w1259]
                tunnel: [w1262] -> _
                tunnel: [w1264] -> w1117
                i -> [w1266]
                stop <- w1262 stop-if-true
                # "Slightly faster version to read data"
                # "Get and display data"
                n483 = Dequeue Element(queue=w1259, timeout in ms (-1)=5000) -> (queue out=w1264:refnum<queue>, element=w1261:cluster{"gain":dbl, bool, "wfm":i16[][]})  [unwired: 1 in, 2 out]
                n484 = Unbundle(w1261) -> ("gain"=w1256:dbl, w1257:bool, "wfm"=w1258:i16[][])
                n485 = case shown="False" w1257 {
                  tunnel: w1258 -> [w1267 w1269]
                  tunnel: [w1267 w1268] -> w1260
                  frame False {
                  }
                  frame True {
                    n486 = call "ReverseData.vi"("Array in"=w1269) -> ("Array out"=w1268:i16[][])
                  }
                }
                n487 = Increment(x=w1266) -> (x+1=w1255:i32)
                n488 = local write "Display index"(w1255) -> ()
                n489 = call "CurrentPlane.vi"("gain"=w1256, "bits A/D"=13, "Axis Vals"=w1265, "Frame"=w1255, "Data"=w1260) -> ("stop out"=w1262:bool)  [unwired: 5 in, 1 out]
                n490 = local write "stop out"(w1262) -> ()
              }
              n491 = global read "MotionGlobals.vi" "DigTimeOut"() -> (w1106)
              n492 = while {
                tunnel: w1086 -> [w1215]
                tunnel: w1126 -> [w1214]
                tunnel: w1085 -> [w1213]
                tunnel: w1095 -> [w1212]
                tunnel: [w1211] -> w1119
                tunnel: w1111 -> [w1209]
                shift-right: [w1207] -> _
                shift-left: w1107 -> [w1208]
                tunnel: [w1206] -> _
                tunnel: w1106 -> [w1205]
                tunnel: "0,1" -> [w1204]
                tunnel: w1092 -> [w1203]
                stop <- w1210 stop-if-true
                n493 = for {
                  tunnel: w1212 -> [w1228]
                  tunnel: w1215 -> [w1230] mode=indexing
                  tunnel: w1204 -> [w1229]
                  tunnel: w1214 -> [w1227]
                  tunnel: [w1223] -> _
                  tunnel: w1213 -> [w1222]
                  tunnel: [w1220] -> w1211
                  tunnel: w1209 -> [w1219]
                  tunnel: w1205 -> [w1218]
                  tunnel: w1203 -> [w1216]
                  i -> [w1217]
                  # "Read data"
                  n494 = case shown="0" w1217 {
                    tunnel: w1230 -> [w1236 w1245]
                    tunnel: w1229 -> [w1234 _]
                    tunnel: w1228 -> [w1237 w1250]
                    tunnel: [w1238 w1249] -> w1226
                    tunnel: [w1231 w1244] -> w1225
                    tunnel: [w1239 w1248] -> w1223
                    tunnel: w1222 -> [w1240 _]
                    tunnel: [w1235 _] -> w1221
                    tunnel: w1219 -> [w1233 _]
                    tunnel: w1218 -> [_ w1246]
                    tunnel: w1216 -> [_ w1242]
                    frame 0 {
                      # "Read files and queue it up."
                      n495 = call <instrlib>:"niScope Initiate Acquisition.vi"("instrument handle"=w1240) -> ("error out"=w1232:errorcluster)  [unwired: 2 in, 12 out]
                      n496 = call "Rapid Read_NI.vi"("NI Card"=w1236, "Channel"=w1234, "Motion Board ID"=w1233, "rf points per line"=w1237, "error in"=w1232) -> ("dig gain"=w1238:dbl, "Array"=w1231:i8[][], "Reverse?"=w1235:bool, "error out"=w1239:errorcluster)  [unwired: 7 in]
                    }
                    frame 1, Default {
                      n497 = property class="niScope"(reference=w1245, "Fetch Record Number"=0, "Fetch Number of Records"=w1242) -> (reference out=w1251:refnum<k15>, error out=w1247:errorcluster)  [unwired: 1 in]
                      n498 = call-poly <instrlib>:"niScope Fetch (poly).vi"("timeout"=w1246, "error in"=w1247, "numSamples"=w1250, "channels"="0", "instrument handle"=w1251) -> ("error out"=w1248:errorcluster, "wfm"=w1244:i8[][], "wfm info"=w1253:T14)  [unwired: 4 out]
                      n499 = Index Array(array=w1253) -> (element=w1252:T15)  [unwired: 1 in]
                      n500 = Unbundle By Name(w1252) -> ("gain"=w1249:dbl)
                    }
                  }
                  n501 = local write "Read Data index"(w1217) -> ()
                  n502 = Bundle("gain"=w1226, "wfm"=w1225, "Reverse?"=w1221, w1217) -> (w1224:T16)  [unwired: 1 in]
                  n503 = Enqueue Element(queue=w1227, element=w1224) -> (queue out=w1220:refnum<queue>)  [unwired: 2 in, 2 out]
                }
                n504 = local read "stop out"() -> (w1210:bool)
                n505 = Tick Count (ms)() -> (millisecond timer value=w1207:u32)
                n506 = Subtract(x=w1207, y=w1208) -> (x-y=w1206:u32)
              }
              n507 = Release Queue(queue=w1119, force destroy? (F)=w1118) -> ()  [unwired: 1 in, 3 out]
              n508 = Release Queue(queue=w1117, force destroy? (F)=w1118) -> ()  [unwired: 1 in, 3 out]
              n509 = Delete Data Value Reference(data value reference=w1094) -> ()  [unwired: 1 in, 2 out]
            }
            frame "Drop Ch 5,4,3" {
              w1298 = 5
              # "Reduced data case that drop ring3,4,5 receive"
              # "Restructure file names"
              # "Read queue and send to files. About same as reading channel by channel"
              n510 = Reshape Array(w1299, w1298, w1298) -> (w1274:T12)
              n511 = expression code="x*5"(w1282) -> (w1277:dbl)
              n512 = Initialize Array(i16 0, w1282, w1273) -> (w1288:i16[][])
              n513 = Index Array(array=w1271) -> (element=w1270)  [unwired: 1 in]
              n514 = Array Subset(array=w1274, length (col)=2 ("index")) -> (w1278:T12)  [unwired: 3 in]
              n515 = Obtain Queue(max queue size (-1, unlimited)=3, element data type=cluster{"gain":dbl, "wfm":i8[][], bool} {"gain"=0.0, "wfm"=[], TRUE}) -> (queue out=w1301:refnum<queue>)  [unwired: 3 in, 2 out]
              n516 = New Data Value Reference(data value=w1288) -> (data value reference=w1287:refnum<data-value>)  [unwired: 1 in, 1 out]
              n517 = Obtain Queue(max queue size (-1, unlimited)=5, element data type=cluster{"gain":dbl, bool, "wfm":i16[][]} {"gain"=0.0, TRUE, "wfm"=[]}) -> (queue out=w1289:refnum<queue>)  [unwired: 3 in, 2 out]
              n518 = Tick Count (ms)() -> (millisecond timer value=w1285:u32)
              n519 = Reshape Array(w1278, 10) -> (w1275:T13)
              n520 = while {
                tunnel: w1270 -> [w1372]
                tunnel: w1301 -> [w1371]
                tunnel: w1277 -> [_]
                tunnel: w1273 -> [w1370]
                tunnel: [w1369] -> w1294
                tunnel: w1286 -> [w1367]
                shift-right: [w1365] -> _
                shift-left: w1285 -> [w1366]
                tunnel: [w1364] -> _
                tunnel: "0,1" -> [w1363]
                i -> [w1358]
                stop <- w1368 stop-if-true
                # "Read files and queue it up."
                # "Read data"
                n521 = local write "Read Data index"(w1358) -> ()
                n522 = call "Rapid Read_NI.vi"("NI Card"=w1372, "Channel"=w1363, "Motion Board ID"=w1367, "rf points per line"=w1370) -> ("dig gain"=w1362:dbl, "Array"=w1361:i8[][], "Reverse?"=w1359:bool)  [unwired: 8 in, 1 out]
                n523 = local read "stop out"() -> (w1368:bool)
                n524 = Bundle("dig gain"=w1362, "Array"=w1361, "Reverse?"=w1359) -> (w1360:T17)  [unwired: 1 in]
                n525 = Tick Count (ms)() -> (millisecond timer value=w1365:u32)
                n526 = Enqueue Element(queue=w1371, element=w1360) -> (queue out=w1369:refnum<queue>)  [unwired: 2 in, 2 out]
                n527 = Subtract(x=w1365, y=w1366) -> (x-y=w1364:u32)
              }
              n528 = while {
                tunnel: w1301 -> [w1324]
                tunnel: w1273 -> [w1323]
                tunnel: [w1319] -> w1293
                tunnel: w1282 -> [w1322]
                tunnel: w1287 -> [w1317]
                tunnel: w1289 -> [w1321]
                tunnel: w1275 -> [w1304]
                shift-right: [w1315] -> _
                shift-left: w1285 -> [w1316]
                tunnel: [w1314] -> _
                tunnel: 10000 -> [w1312]
                tunnel: i16[] [1, 1, 1, 1, 2, 2, 2, 2, 2, 2] -> [w1311]
                tunnel: 10 -> [w1305]
                tunnel: [w1303] -> w1272
                i -> [w1318]
                stop <- w1319 stop-if-true
                n529 = Dequeue Element(queue=w1324, timeout in ms (-1)=w1312) -> (element=w1310:cluster{"gain":dbl, "wfm":i8[][], bool})  [unwired: 1 in, 3 out]
                n530 = local write "SF Index"(w1318) -> ()
                n531 = Unbundle(w1310) -> ("gain"=w1320:dbl, "wfm"=w1309:i8[][], w1306:bool)
                n532 = Multiply(x=w1323, y=w1305) -> (x*y=w1307:i32)
                n533 = Reshape Array(w1309, w1322, w1307) -> (w1308:i8[][])
                n534 = for {
                  N: w1305 -> [_]
                  tunnel: w1304 -> [w1332]
                  tunnel: [w1335] -> w1313
                  tunnel: w1317 -> [w1334]
                  shift-right: [w1327] -> _
                  shift-left: w1308 -> [w1337]
                  tunnel: w1323 -> [w1326]
                  tunnel: w1311 -> [w1325] mode=indexing
                  i -> [w1333]
                  n535 = Index Array(array=w1332, index=w1333) -> (element=w1331:T11)
                  n536 = Delete From Array(array=w1337, length=w1326, index (col)=0 ("disabled index (col)")) -> (deleted portion=w1330:i8[], array with subset deleted=w1327:i8[][])  [unwired: 1 in]
                  n537 = for {
                    tunnel: w1330 -> [w1340] mode=indexing
                    tunnel: [w1339] -> w1329 mode=indexing
                    n538 = call-poly <vilib>:"Mean.vi"("X"=w1340) -> ("mean"=w1341:dbl)  [unwired: 1 out]
                    n539 = To Word Integer(number=w1341) -> (16bit integer=w1338:i16)
                    n540 = Subtract(x=w1340, y=w1338) -> (x-y=w1339:i16)
                  }
                  n541 = call-poly "TimeShiftDataPoly.vi"("output cluster"=w1331, "Array In"=w1329) -> ("Array Out"=w1336:i16[][])  [unwired: 2 in]
                  n542 = in-place {
                    in-place-border: w1336 -> [w1343]
                    in-place-border: w1325 -> [w1344]
                    n543 = in-place-dvr #7(w1334) -> (w1345:i16[][])  [unwired: 1 out]
                    n544 = case shown="2" w1344 {
                      selector: w1344 -> [_ w1348]
                      tunnel: w1343 -> [w1347 w1350]
                      tunnel: [w1347 w1349] -> w1342
                      frame 0, Default {
                      }
                      frame 2 {
                        n545 = Multiply(x=w1348, y=w1350) -> (x*y=w1349:i16[][])
                      }
                    }
                    n546 = Add(x=w1342, y=w1345) -> (x+y=w1346:i16[][])
                    n547 = in-place-dvr #7(w1346) -> (w1335:refnum<data-value>)  [unwired: 1 out]
                  }
                }
                n548 = local read "stop out"() -> (w1319:bool)
                n549 = in-place {
                  in-place-border: w1321 -> [w1357]
                  in-place-border: w1306 -> [w1356]
                  in-place-border: w1320 -> [w1355]
                  n550 = in-place-dvr #8(w1313) -> (w1351:i16[][])  [unwired: 1 out]
                  n551 = Bundle("gain"=w1355, w1356, w1351) -> (w1354:cluster{"gain":dbl, bool, i16[][]})  [unwired: 1 in]
                  n552 = Multiply(x=i16 0, y=w1351) -> (x*y=w1353:i16[][])
                  n553 = Enqueue Element(queue=w1357, element=w1354) -> ()  [unwired: 2 in, 3 out]
                  n554 = in-place-dvr #8(w1353) -> (w1303:refnum<data-value>)  [unwired: 1 out]
                }
                n555 = Tick Count (ms)() -> (millisecond timer value=w1315:u32)
                n556 = Subtract(x=w1315, y=w1316) -> (x-y=w1314:u32)
              }
              n557 = while {
                tunnel: w1291 -> [w1384]
                tunnel: w1289 -> [w1378]
                tunnel: [w1381] -> _
                tunnel: [w1383] -> w1292
                i -> [w1385]
                stop <- w1381 stop-if-true
                # "Slightly faster version to read data"
                # "Get and display data"
                n558 = Dequeue Element(queue=w1378, timeout in ms (-1)=5000) -> (queue out=w1383:refnum<queue>, element=w1380:cluster{"gain":dbl, bool, "wfm":i16[][]})  [unwired: 1 in, 2 out]
                n559 = Unbundle(w1380) -> ("gain"=w1375:dbl, w1376:bool, "wfm"=w1377:i16[][])
                n560 = case shown="False" w1376 {
                  tunnel: w1377 -> [w1386 w1388]
                  tunnel: [w1386 w1387] -> w1379
                  frame False {
                  }
                  frame True {
                    n561 = call "ReverseData.vi"("Array in"=w1388) -> ("Array out"=w1387:i16[][])
                  }
                }
                n562 = Increment(x=w1385) -> (x+1=w1374:i32)
                n563 = local write "Display index"(w1374) -> ()
                n564 = call "CurrentPlane.vi"("gain"=w1375, "bits A/D"=13, "Axis Vals"=w1384, "Frame"=w1374, "Data"=w1379) -> ("stop out"=w1381:bool)  [unwired: 5 in, 1 out]
                n565 = local write "stop out"(w1381) -> ()
              }
              n566 = Release Queue(queue=w1294, force destroy? (F)=w1293) -> ()  [unwired: 1 in, 3 out]
              n567 = Release Queue(queue=w1292, force destroy? (F)=w1293) -> ()  [unwired: 1 in, 3 out]
              n568 = Delete Data Value Reference(data value reference=w1272) -> ()  [unwired: 1 in, 2 out]
            }
            frame "All 25 FIFO CH by CH" {
              w1414 = 5
              w1398 = "1"
              # "Read queue and send to files."
              n569 = Interleave 1D Arrays(w1390, w1390) -> (w1394:dbl[])
              n570 = Index Array(array=w1390, index=2) -> (element=w1389)
              n571 = Index Array(array=w1390, index=1) -> (element=w1391)
              n572 = expression code="x*5"(w1404) -> (w1416:dbl)
              n573 = Reshape Array(w1415, w1414, w1414) -> (w1413:T12)
              n574 = Initialize Array(i16 0, w1404, w1397) -> (w1402:i16[][])
              n575 = Obtain Queue(max queue size (-1, unlimited)=25, element data type=T9 {"gain"=0.0, "wfm"=[], TRUE, "max queue size (-1, unlimited)"=25}) -> (queue out=w1420:refnum<queue>)  [unwired: 3 in, 2 out]
              n576 = New Data Value Reference(data value=w1402) -> (data value reference=w1401:refnum<data-value>)  [unwired: 1 in, 1 out]
              n577 = expression code="x*5"(w1397) -> (w1418:dbl)
              n578 = Obtain Queue(max queue size (-1, unlimited)=5, element data type=cluster{"gain":dbl, bool, "wfm":i16[][]} {"gain"=0.0, TRUE, "wfm"=[]}) -> (queue out=w1403:refnum<queue>)  [unwired: 3 in, 2 out]
              n579 = Tick Count (ms)() -> (millisecond timer value=w1399:u32)
              n580 = Build Array("0", w1398, "0", w1398, w1398) -> (w1422:string[])
              n581 = while {
                tunnel: w1422 -> [w1491]
                tunnel: w1420 -> [w1490]
                tunnel: w1391 -> [w1489]
                tunnel: w1389 -> [w1488]
                tunnel: w1416 -> [w1487]
                tunnel: w1397 -> [w1486]
                tunnel: [w1485] -> w1409
                tunnel: w1400 -> [w1483]
                shift-right: [w1481] -> _
                shift-left: w1399 -> [w1482]
                tunnel: [w1480] -> _
                tunnel: w1394 -> [w1479]
                stop <- w1484 stop-if-true
                n582 = for {
                  tunnel: w1486 -> [w1503]
                  tunnel: w1487 -> [w1506]
                  tunnel: w1479 -> [w1505] mode=indexing
                  tunnel: w1491 -> [w1504] mode=indexing
                  tunnel: w1490 -> [w1502]
                  tunnel: [w1498] -> _
                  tunnel: w1489 -> [w1497]
                  tunnel: w1488 -> [w1496]
                  tunnel: [w1494] -> w1485
                  tunnel: w1483 -> [w1493]
                  i -> [w1492]
                  # "Read data"
                  n583 = case shown="0" w1492 {
                    tunnel: w1506 -> [_ w1528]
                    tunnel: w1505 -> [w1510 w1527]
                    tunnel: w1504 -> [w1508 w1525]
                    tunnel: w1503 -> [w1511 w1524]
                    tunnel: [w1512 w1523] -> w1501
                    tunnel: [w1514 w1522] -> w1500
                    tunnel: [w1513 w1521] -> w1498
                    tunnel: w1497 -> [w1518 _]
                    tunnel: w1496 -> [w1517 _]
                    tunnel: [w1509 _] -> w1495
                    tunnel: w1493 -> [w1507 _]
                    frame 0 {
                      # "Read files and queue it up."
                      n584 = call <instrlib>:"niScope Initiate Acquisition.vi"("instrument handle"=w1518) -> ("error out"=w1516:errorcluster)  [unwired: 2 in, 12 out]
                      n585 = call <instrlib>:"niScope Initiate Acquisition.vi"("instrument handle"=w1517, "error in"=w1516) -> ("error out"=w1515:errorcluster)  [unwired: 1 in, 12 out]
                      n586 = call "Rapid Read_NI.vi"("NI Card"=w1510, "Channel"=w1508, "Motion Board ID"=w1507, "rf points per line"=w1511, "error in"=w1515) -> ("dig gain"=w1512:dbl, "Array"=w1514:i8[][], "Reverse?"=w1509:bool, "error out"=w1513:errorcluster)  [unwired: 7 in]
                    }
                    frame 1, Default {
                      n587 = property class="niScope"(reference=w1527, "Fetch Record Number"=0, "Fetch Number of Records"=w1528) -> (reference out=w1526:refnum<k15>, error out=w1520:errorcluster)  [unwired: 1 in]
                      n588 = call-poly <instrlib>:"niScope Fetch (poly).vi"("timeout"=0.0, "error in"=w1520, "numSamples"=w1524, "channels"=w1525, "instrument handle"=w1526) -> ("error out"=w1521:errorcluster, "wfm"=w1522:i8[][], "wfm info"=w1531:T14)  [unwired: 4 out]
                      n589 = Index Array(array=w1531) -> (element=w1530:T15)  [unwired: 1 in]
                      n590 = Unbundle By Name(w1530) -> ("gain"=w1523:dbl)
                    }
                  }
                  n591 = local write "Read Data index"(w1492) -> ()
                  n592 = Bundle("gain"=w1501, "wfm"=w1500, "Reverse?"=w1495, w1492) -> (w1499:T16)  [unwired: 1 in]
                  n593 = Enqueue Element(queue=w1502, element=w1499) -> (queue out=w1494:refnum<queue>)  [unwired: 2 in, 2 out]
                }
                n594 = local read "stop out"() -> (w1484:bool)
                n595 = Tick Count (ms)() -> (millisecond timer value=w1481:u32)
                n596 = Subtract(x=w1481, y=w1482) -> (x-y=w1480:u32)
              }
              n597 = while {
                tunnel: w1420 -> [w1439]
                tunnel: w1418 -> [w1438]
                tunnel: w1413 -> [w1426]
                tunnel: [w1434] -> w1408
                tunnel: w1404 -> [w1437]
                tunnel: w1401 -> [w1432]
                tunnel: w1403 -> [w1436]
                shift-right: [w1429] -> _
                shift-left: w1399 -> [w1430]
                tunnel: [w1428] -> _
                tunnel: w1397 -> [w1427]
                tunnel: [w1423] -> w1396
                i -> [w1433]
                stop <- w1434 stop-if-true
                n598 = for {
                  tunnel: w1438 -> [w1461]
                  tunnel: w1437 -> [w1455]
                  tunnel: w1439 -> [w1460]
                  tunnel: w1426 -> [_] mode=indexing
                  tunnel: [w1454] -> w1424 mode=indexing
                  tunnel: [w1453] -> w1435
                  tunnel: [w1452] -> w1431
                  tunnel: w1432 -> [w1451]
                  tunnel: w1427 -> [w1450]
                  tunnel: w1426 -> [w1449]
                  workers-P: _ -> [_]
                  n599 = Dequeue Element(queue=w1460, timeout in ms (-1)=10000) -> (element=w1459:T9)  [unwired: 1 in, 3 out]
                  n600 = Unbundle(w1459) -> ("gain"=w1453:dbl, "wfm"=w1458:i8[][], w1454:bool, "max queue size (-1, unlimited)"=w1447:i32)
                  n601 = Index Array(array=w1449, index (row)=w1447) -> (element=w1448:T13)  [unwired: 1 in]
                  n602 = Reshape Array(w1458, w1455, w1461) -> (w1457:i8[][])
                  n603 = for {
                    tunnel: w1448 -> [w1470] mode=indexing
                    tunnel: [w1468] -> w1452
                    tunnel: w1451 -> [w1467]
                    tunnel: w1450 -> [w1463]
                    shift-right: [w1462] -> _
                    shift-left: w1457 -> [w1471]
                    n604 = Delete From Array(array=w1471, length=w1463, index (col)=0 ("disabled index (col)")) -> (deleted portion=w1466:i8[], array with subset deleted=w1462:i8[][])  [unwired: 1 in]
                    n605 = for {
                      tunnel: w1466 -> [w1474] mode=indexing
                      tunnel: [w1473] -> w1465 mode=indexing
                      n606 = call-poly <vilib>:"Mean.vi"("X"=w1474) -> ("mean"=w1475:dbl)  [unwired: 1 out]
                      n607 = To Word Integer(number=w1475) -> (16bit integer=w1472:i16)
                      n608 = Subtract(x=w1474, y=w1472) -> (x-y=w1473:i16)
                    }
                    n609 = call-poly "TimeShiftDataPoly.vi"("output cluster"=w1470, "Array In"=w1465) -> ("Array Out"=w1469:i16[][])  [unwired: 2 in]
                    n610 = in-place {
                      in-place-border: w1469 -> [w1478]
                      n611 = in-place-dvr #9(w1467) -> (w1476:i16[][])  [unwired: 1 out]
                      n612 = Add(x=w1478, y=w1476) -> (x+y=w1477:i16[][])
                      n613 = in-place-dvr #9(w1477) -> (w1468:refnum<data-value>)  [unwired: 1 out]
                    }
                  }
                }
                n614 = local write "SF Index"(w1433) -> ()
                n615 = local read "stop out"() -> (w1434:bool)
                n616 = Or Array Elements(Boolean array=w1424) -> (logical OR=w1425:bool)
                n617 = in-place {
                  in-place-border: w1436 -> [w1446]
                  in-place-border: w1425 -> [w1445]
                  in-place-border: w1435 -> [w1444]
                  n618 = in-place-dvr #10(w1431) -> (w1440:i16[][])  [unwired: 1 out]
                  n619 = Bundle("gain"=w1444, w1445, w1440) -> (w1443:cluster{"gain":dbl, bool, i16[][]})  [unwired: 1 in]
                  n620 = Multiply(x=i16 0, y=w1440) -> (x*y=w1442:i16[][])
                  n621 = Enqueue Element(queue=w1446, element=w1443) -> ()  [unwired: 2 in, 3 out]
                  n622 = in-place-dvr #10(w1442) -> (w1423:refnum<data-value>)  [unwired: 1 out]
                }
                n623 = Tick Count (ms)() -> (millisecond timer value=w1429:u32)
                n624 = Subtract(x=w1429, y=w1430) -> (x-y=w1428:u32)
              }
              n625 = while {
                tunnel: w1406 -> [w1543]
                tunnel: w1403 -> [w1537]
                tunnel: [w1540] -> _
                tunnel: [w1542] -> w1407
                i -> [w1544]
                stop <- w1540 stop-if-true
                # "Slightly faster version to read data"
                # "Get and display data"
                n626 = Dequeue Element(queue=w1537, timeout in ms (-1)=5000) -> (queue out=w1542:refnum<queue>, element=w1539:cluster{"gain":dbl, bool, "wfm":i16[][]})  [unwired: 1 in, 2 out]
                n627 = Unbundle(w1539) -> ("gain"=w1534:dbl, w1535:bool, "wfm"=w1536:i16[][])
                n628 = case shown="True" w1535 {
                  tunnel: w1536 -> [w1545 w1547]
                  tunnel: [w1545 w1546] -> w1538
                  frame False {
                  }
                  frame True {
                    n629 = call "ReverseData.vi"("Array in"=w1547) -> ("Array out"=w1546:i16[][])
                  }
                }
                n630 = Increment(x=w1544) -> (x+1=w1533:i32)
                n631 = local write "Display index"(w1533) -> ()
                n632 = call "CurrentPlane.vi"("gain"=w1534, "bits A/D"=13, "Axis Vals"=w1543, "Frame"=w1533, "Data"=w1538) -> ("stop out"=w1540:bool)  [unwired: 5 in, 1 out]
                n633 = local write "stop out"(w1540) -> ()
              }
              n634 = Delete Data Value Reference(data value reference=w1396) -> ()  [unwired: 1 in, 2 out]
              n635 = Release Queue(queue=w1409, force destroy? (F)=w1408) -> ()  [unwired: 1 in, 3 out]
              n636 = Release Queue(queue=w1407, force destroy? (F)=w1408) -> ()  [unwired: 1 in, 3 out]
            }
            frame "Line by line 2 Ch" {
              w1559 = 5
              # "Not fast enough for read"
              # "Read queue and send to files for chans 1,2"
              n637 = Reshape Array(w1554, w1559, w1559) -> (w1555:T12)
              n638 = Initialize Array(i16 0, w1564, w1551) -> (w1566:i16[][])
              n639 = Index Array(array=w1549) -> (element=w1548)  [unwired: 1 in]
              n640 = Array Subset(array=w1555, length (col)=2 ("index")) -> (w1556:T12)  [unwired: 3 in]
              n641 = Obtain Queue(max queue size (-1, unlimited)=30, element data type=cluster{"gain":dbl, "wfm":i8[][], bool} {"gain"=0.0, "wfm"=[], TRUE}) -> (queue out=w1561:refnum<queue>)  [unwired: 3 in, 2 out]
              n642 = New Data Value Reference(data value=w1566) -> (data value reference=w1565:refnum<data-value>)  [unwired: 1 in, 1 out]
              n643 = Reshape Array(w1556, 10) -> (w1553:T13)
              n644 = Obtain Queue(max queue size (-1, unlimited)=3, element data type=cluster{"gain":dbl, bool, "wfm":i16[][]} {"gain"=0.0, TRUE, "wfm"=[]}) -> (queue out=w1567:refnum<queue>)  [unwired: 3 in, 2 out]
              n645 = Tick Count (ms)() -> (millisecond timer value=w1560:u32)
              n646 = while {
                tunnel: w1564 -> [w1625]
                tunnel: w1551 -> [w1624]
                tunnel: w1563 -> [w1621]
                tunnel: w1561 -> [w1620]
                shift-right: [w1616] -> _
                shift-left: w1560 -> [w1618]
                tunnel: [w1617] -> _
                tunnel: w1548 -> [w1615]
                i -> [w1622]
                stop <- w1623 stop-if-true
                # "Read files and queue it up."
                # "Read data"
                n647 = local write "Read Data index"(w1622) -> ()
                n648 = call "Rapid Read_2Ch.vi"("NI Card 3"=w1615, "Motion Board ID"=w1621, "rf points per line"=w1624, "lines per plane"=w1625, "queue out"=w1620) -> ("error out"=w1619:errorcluster)  [unwired: 7 in, 3 out]
                n649 = flat-sequence {
                  tunnel: w1619 -> [_]
                  tunnel: [w1626] -> w1616
                  frame #0 {
                    n650 = Tick Count (ms)() -> (millisecond timer value=w1626:u32)
                  }
                }
                n651 = local read "stop out"() -> (w1623:bool)
                n652 = Subtract(x=w1616, y=w1618) -> (x-y=w1617:u32)
              }
              n653 = while {
                tunnel: w1561 -> [w1579]
                tunnel: w1553 -> [w1587]
                tunnel: [w1583] -> w1571
                tunnel: w1565 -> [w1581]
                tunnel: w1567 -> [w1586]
                tunnel: [w1579] -> w1562
                tunnel: i16[] [1, 1, 1, 1, 2, 2, 2, 2, 2, 2] -> [w1578]
                tunnel: [w1577] -> w1550
                i -> [w1582]
                stop <- w1583 stop-if-true
                n654 = for {
                  tunnel: w1579 -> [w1605]
                  tunnel: w1587 -> [w1597] mode=indexing
                  tunnel: [w1602] -> w1585
                  tunnel: [w1601] -> w1584
                  tunnel: [w1600] -> w1580
                  tunnel: w1581 -> [w1599]
                  tunnel: w1578 -> [w1595] mode=indexing
                  n655 = Dequeue Element(queue=w1605, timeout in ms (-1)=10000) -> (element=w1604:cluster{"gain":dbl, "wfm":i8[][], bool})  [unwired: 1 in, 3 out]
                  n656 = Unbundle(w1604) -> ("gain"=w1601:dbl, "wfm"=w1596:i8[][], w1602:bool)
                  n657 = call-poly "TimeShiftDataPoly.vi"("output cluster"=w1597, "Array In"=w1596) -> ("Array Out"=w1598:i8[][])  [unwired: 1 in, 1 out]
                  n658 = in-place {
                    in-place-border: w1598 -> [w1607]
                    in-place-border: w1595 -> [w1608]
                    n659 = in-place-dvr #11(w1599) -> (w1609:i16[][])  [unwired: 1 out]
                    n660 = case shown="2" w1608 {
                      selector: w1608 -> [_ w1612]
                      tunnel: w1607 -> [w1611 w1614]
                      tunnel: [w1611 w1613] -> w1606
                      frame 0, Default {
                      }
                      frame 2 {
                        n661 = Multiply(x=w1612, y=w1614) -> (x*y=w1613:i16[][])
                      }
                    }
                    n662 = Add(x=w1606, y=w1609) -> (x+y=w1610:i16[][])
                    n663 = in-place-dvr #11(w1610) -> (w1600:refnum<data-value>)  [unwired: 1 out]
                  }
                }
                n664 = local write "SF Index"(w1582) -> ()
                n665 = local read "stop out"() -> (w1583:bool)
                n666 = in-place {
                  in-place-border: w1586 -> [w1594]
                  in-place-border: w1585 -> [w1593]
                  in-place-border: w1584 -> [w1592]
                  n667 = in-place-dvr #12(w1580) -> (w1588:i16[][])  [unwired: 1 out]
                  n668 = Bundle("gain"=w1592, w1593, w1588) -> (w1591:cluster{"gain":dbl, bool, i16[][]})  [unwired: 1 in]
                  n669 = Multiply(x=i16 0, y=w1588) -> (x*y=w1590:i16[][])
                  n670 = Enqueue Element(queue=w1594, element=w1591) -> ()  [unwired: 2 in, 3 out]
                  n671 = in-place-dvr #12(w1590) -> (w1577:refnum<data-value>)  [unwired: 1 out]
                }
              }
              n672 = while {
                tunnel: w1569 -> [w1638]
                tunnel: w1567 -> [w1632]
                tunnel: [w1635] -> _
                tunnel: [w1637] -> w1570
                i -> [w1639]
                stop <- w1635 stop-if-true
                # "Slightly faster version to read data"
                # "Get and display data"
                n673 = Dequeue Element(queue=w1632, timeout in ms (-1)=3000) -> (queue out=w1637:refnum<queue>, element=w1634:cluster{"gain":dbl, bool, "wfm":i16[][]})  [unwired: 1 in, 2 out]
                n674 = Unbundle(w1634) -> ("gain"=w1629:dbl, w1630:bool, "wfm"=w1631:i16[][])
                n675 = case shown="True" w1630 {
                  tunnel: w1631 -> [w1640 w1642]
                  tunnel: [w1640 w1641] -> w1633
                  frame False {
                  }
                  frame True {
                    n676 = call "ReverseData.vi"("Array in"=w1642) -> ("Array out"=w1641:i16[][])
                  }
                }
                n677 = Increment(x=w1639) -> (x+1=w1628:i32)
                n678 = local write "Display index"(w1628) -> ()
                n679 = call "CurrentPlane.vi"("gain"=w1629, "bits A/D"=13, "Axis Vals"=w1638, "Frame"=w1628, "Data"=w1633) -> ("stop out"=w1635:bool)  [unwired: 5 in, 1 out]
                n680 = local write "stop out"(w1635) -> ()
              }
              n681 = Release Queue(queue=w1570, force destroy? (F)=w1571) -> ()  [unwired: 1 in, 3 out]
              n682 = Delete Data Value Reference(data value reference=w1550) -> ()  [unwired: 1 in, 2 out]
              n683 = Release Queue(queue=w1562, force destroy? (F)=w1571) -> ()  [unwired: 1 in, 3 out]
            }
            frame "Line by line All" {
              # "Not fast enough for read"
              # "Read queue and send to files all 25"
              n684 = global read "MotionGlobals.vi" "rf points per line"() -> (w1654)
              n685 = Initialize Array(i16 0, w1649, w1654) -> (w1652:i16[][])
              n686 = Obtain Queue(max queue size (-1, unlimited)=75, element data type=T9 {"gain"=0.0, "wfm"=[], TRUE, "max queue size (-1, unlimited)"=1}) -> (queue out=w1646:refnum<queue>)  [unwired: 3 in, 2 out]
              n687 = New Data Value Reference(data value=w1652) -> (data value reference=w1651:refnum<data-value>)  [unwired: 1 in, 1 out]
              n688 = Tick Count (ms)() -> (millisecond timer value=w1645:u32)
              n689 = Obtain Queue(max queue size (-1, unlimited)=3, element data type=cluster{"gain":dbl, bool, "wfm":i16[][]} {"gain"=0.0, TRUE, "wfm"=[]}) -> (queue out=w1653:refnum<queue>)  [unwired: 3 in, 2 out]
              n690 = while {
                tunnel: w1649 -> [w1707]
                tunnel: w1662 -> [w1706]
                tunnel: w1643 -> [w1703]
                tunnel: w1648 -> [w1702]
                tunnel: w1646 -> [w1701]
                tunnel: [w1700] -> _
                shift-right: [w1697] -> _
                shift-left: w1645 -> [w1699]
                tunnel: [w1698] -> _
                i -> [w1704]
                stop <- w1705 stop-if-true
                # "Read files and queue it up."
                # "Read data"
                n691 = local write "Read Data index"(w1704) -> ()
                n692 = call "Rapid Read_5Ch.vi"("Dig Cards"=w1703, "Motion Board ID"=w1702, "rf points per line"=w1706, "lines per plane"=w1707, "queue out"=w1701) -> ("error out"=w1700:errorcluster)  [unwired: 7 in, 3 out]
                n693 = flat-sequence {
                  tunnel: w1700 -> [_]
                  tunnel: [w1708] -> w1697
                  frame #0 {
                    n694 = Tick Count (ms)() -> (millisecond timer value=w1708:u32)
                  }
                }
                n695 = local read "stop out"() -> (w1705:bool)
                n696 = Subtract(x=w1697, y=w1699) -> (x-y=w1698:u32)
              }
              n697 = while {
                tunnel: w1646 -> [w1667]
                tunnel: w1650 -> [w1665]
                tunnel: [w1671] -> w1658
                tunnel: w1651 -> [w1669]
                tunnel: w1653 -> [w1674]
                tunnel: [w1667] -> w1647
                tunnel: [w1666] -> w1644
                i -> [w1670]
                stop <- w1671 stop-if-true
                n698 = for {
                  tunnel: w1667 -> [w1693]
                  tunnel: w1665 -> [_] mode=indexing
                  tunnel: [w1690] -> w1673
                  tunnel: [w1689] -> w1672
                  tunnel: [w1688] -> w1668
                  tunnel: w1669 -> [w1687]
                  tunnel: w1665 -> [w1684]
                  n699 = Dequeue Element(queue=w1693, timeout in ms (-1)=10000) -> (element=w1692:T9)  [unwired: 1 in, 3 out]
                  n700 = Unbundle(w1692) -> ("gain"=w1689:dbl, "wfm"=w1685:i8[][], w1690:bool, "max queue size (-1, unlimited)"=w1683:i32)
                  n701 = Index Array(array=w1684, index=w1683) -> (element=w1682:T11)
                  n702 = call-poly "TimeShiftDataPoly.vi"("output cluster"=w1682, "Array In"=w1685) -> ("Array Out"=w1686:i8[][])  [unwired: 1 in, 1 out]
                  n703 = in-place {
                    in-place-border: w1686 -> [w1696]
                    n704 = in-place-dvr #13(w1687) -> (w1694:i16[][])  [unwired: 1 out]
                    n705 = Add(x=w1696, y=w1694) -> (x+y=w1695:i16[][])
                    n706 = in-place-dvr #13(w1695) -> (w1688:refnum<data-value>)  [unwired: 1 out]
                  }
                }
                n707 = local write "SF Index"(w1670) -> ()
                n708 = local read "stop out"() -> (w1671:bool)
                n709 = in-place {
                  in-place-border: w1674 -> [w1681]
                  in-place-border: w1673 -> [w1680]
                  in-place-border: w1672 -> [w1679]
                  n710 = in-place-dvr #14(w1668) -> (w1675:i16[][])  [unwired: 1 out]
                  n711 = Bundle("gain"=w1679, w1680, w1675) -> (w1678:cluster{"gain":dbl, bool, i16[][]})  [unwired: 1 in]
                  n712 = Multiply(x=i16 0, y=w1675) -> (x*y=w1677:i16[][])
                  n713 = Enqueue Element(queue=w1681, element=w1678) -> ()  [unwired: 2 in, 3 out]
                  n714 = in-place-dvr #14(w1677) -> (w1666:refnum<data-value>)  [unwired: 1 out]
                }
              }
              n715 = while {
                tunnel: w1656 -> [w1720]
                tunnel: w1653 -> [w1714]
                tunnel: [w1717] -> _
                tunnel: [w1719] -> w1657
                i -> [w1721]
                stop <- w1717 stop-if-true
                # "Slightly faster version to read data"
                # "Get and display data"
                n716 = Dequeue Element(queue=w1714, timeout in ms (-1)=3000) -> (queue out=w1719:refnum<queue>, element=w1716:cluster{"gain":dbl, bool, "wfm":i16[][]})  [unwired: 1 in, 2 out]
                n717 = Unbundle(w1716) -> ("gain"=w1711:dbl, w1712:bool, "wfm"=w1713:i16[][])
                n718 = case shown="True" w1712 {
                  tunnel: w1713 -> [w1722 w1724]
                  tunnel: [w1722 w1723] -> w1715
                  frame False {
                  }
                  frame True {
                    n719 = call "ReverseData.vi"("Array in"=w1724) -> ("Array out"=w1723:i16[][])
                  }
                }
                n720 = Increment(x=w1721) -> (x+1=w1710:i32)
                n721 = local write "Display index"(w1710) -> ()
                n722 = call "CurrentPlane.vi"("gain"=w1711, "bits A/D"=13, "Axis Vals"=w1720, "Frame"=w1710, "Data"=w1715) -> ("stop out"=w1717:bool)  [unwired: 5 in, 1 out]
                n723 = local write "stop out"(w1717) -> ()
              }
              n724 = Release Queue(queue=w1647, force destroy? (F)=w1658) -> ()  [unwired: 1 in, 3 out]
              n725 = Release Queue(queue=w1657, force destroy? (F)=w1658) -> ()  [unwired: 1 in, 3 out]
              n726 = Delete Data Value Reference(data value reference=w1644) -> ()  [unwired: 1 in, 2 out]
            }
            frame "Deep Memory 2 CH" {
              w1748 = 5
              # "Just Ch 1,2. Also cam suffer memory overflow if Byte depth too small"
              # "Arm digitizer"
              n727 = Index Array(array=w1726) -> (element=w1725)  [unwired: 1 in]
              n728 = Reshape Array(w1743, w1748, w1748) -> (w1744:T12)
              n729 = call <instrlib>:"niScope Initiate Acquisition.vi"("instrument handle"=w1725) -> ("error out"=w1730:errorcluster)  [unwired: 2 in, 12 out]
              n730 = expression code="x*5"(w1734) -> (w1749:dbl)
              n731 = Initialize Array(i16 0, w1734, w1737) -> (w1756:i16[][])
              n732 = Array Subset(array=w1744, length (col)=2 ("index")) -> (w1745:T12)  [unwired: 3 in]
              n733 = Tick Count (ms)() -> (millisecond timer value=w1727:u32)
              n734 = Obtain Queue(max queue size (-1, unlimited)=5, element data type=cluster{"Fetch:Records Done":i32, bool} {"Fetch:Records Done"=0, TRUE}) -> (queue out=w1728:refnum<queue>)  [unwired: 2 in, 3 out]
              n735 = node-c288(i64 50 ("Period")) -> (w1759:T6)
              n736 = Obtain Queue(max queue size (-1, unlimited)=5, element data type=i8[][] [] ("Array")) -> (queue out=w1742:refnum<queue>)  [unwired: 2 in, 3 out]
              n737 = New Data Value Reference(data value=w1756) -> (data value reference=w1740:refnum<data-value>)  [unwired: 1 in, 1 out]
              n738 = Tick Count (ms)() -> (millisecond timer value=w1736:u32)
              n739 = Obtain Queue(max queue size (-1, unlimited)=5, element data type=i16[][] [] ("wfm")) -> (queue out=w1741:refnum<queue>)  [unwired: 3 in, 2 out]
              n740 = Reshape Array(w1745, 10) -> (w1739:T13)
              n741 = while {
                tunnel: w1728 -> [w1888]
                tunnel: [w1897] -> w1765
                tunnel: w1725 -> [w1898]
                tunnel: w1742 -> [w1900]
                tunnel: w1737 -> [w1889]
                tunnel: [w1884] -> w1763
                tunnel: w1730 -> [w1896]
                tunnel: w1749 -> [w1885]
                tunnel: [w1882] -> w1731
                shift-right: [w1881] -> _
                shift-left: w1727 -> [w1880]
                tunnel: [w1878] -> _
                i -> [w1891]
                stop <- w1897 stop-if-true
                # "This loop reads the data once it is in the queue"
                # "Get and display data"
                n742 = Dequeue Element(queue=w1888, timeout in ms (-1)=1000, error in (no error)=w1896) -> (queue out=w1887:refnum<queue>, element=w1901:cluster{"Fetch:Records Done":i32, bool}, error out=w1892:errorcluster)  [unwired: 1 out]
                n743 = Unbundle(w1901) -> ("Fetch:Records Done"=w1894:i32)  [unwired: 1 out]
                n744 = local write "Read Data index"(w1891) -> ()
                n745 = property class="niScope"(reference=w1898, error in=w1892, "Fetch Record Number"=w1894, "Fetch Number of Records"=w1885) -> (reference out=w1890:refnum<k15>, error out=w1893:errorcluster)
                n746 = call-poly <instrlib>:"niScope Fetch (poly).vi"("timeout"=3.0, "error in"=w1893, "numSamples"=w1889, "channels"="0,1", "instrument handle"=w1890) -> ("error out"=w1879:errorcluster, "wfm"=w1895:i8[][], "instrument handle out"=w1882:refnum<k15>)  [unwired: 4 out]
                n747 = case shown="No Error" w1879 {
                  tunnel: w1900 -> [w1908 w1909]
                  tunnel: w1895 -> [w1907 _]
                  tunnel: w1887 -> [w1906 _]
                  tunnel: [w1905 w1909] -> w1884
                  frame No Error {
                    n748 = Lossy Enqueue Element(queue=w1908, element=w1907) -> (queue out=w1905:refnum<queue>, error out=w1904:errorcluster)  [unwired: 1 in, 2 out]
                    n749 = Get Queue Status(queue=w1906, error in (no error)=w1904) -> (# elements in queue=w1903:i32)  [unwired: 1 in, 7 out]
                    n750 = local write "SF queue"(w1903) -> ()
                  }
                  frame Error {
                  }
                }
                n751 = stacked-sequence {
                  tunnel: [w1902] -> w1881
                  tunnel: w1879 -> [_]
                  frame #0 {
                    n752 = Tick Count (ms)() -> (millisecond timer value=w1902:u32)
                  }
                }
                n753 = Subtract(x=w1881, y=w1880) -> (x-y=w1878:u32)
                n754 = local read "stop out"() -> (w1897:bool)
              }
              n755 = timed-loop {
                shift-right: [w1846] -> _
                shift-left: 0 -> [w1853]
                shift-right: [w1859] -> _
                shift-left: TRUE -> [w1854]
                tunnel: w1768 -> [w1857]
                tunnel: [w1852] -> w1760
                tunnel: [w1842] -> w1764
                tunnel: w1725 -> [w1851]
                tunnel: w1761 -> [w1847]
                tunnel: w1730 -> [w1856]
                timing: w1759 -> [_]
                timing-out: [_] -> w1758
                tunnel: w1728 -> [w1839]
                i -> [w1841]
                stop <- w1852 stop-if-true
                # "This loop performs back and forth scan and records record # at end of run"
                n756 = Bundle(w1853, w1854) -> (w1850:cluster{i32, bool})  [unwired: 1 in]
                n757 = Select(t=T5 6 ("Program (1)"), s=w1854, f=T5 7 ("Program (1)")) -> (s? t:f=w1840:T5)
                n758 = call <vilib>:"Run Program.flx"("error in (no error)"=w1856, "Program (1)"=w1840, "Board ID"=w1857) -> ("error out"=w1849:errorcluster, "Bd ID Out"=w1844:T2)  [unwired: 4 out]
                n759 = stacked-sequence {
                  tunnel: w1849 -> [w1871]
                  tunnel: [w1871] -> w1848
                  tunnel: [w1869] -> w1845
                  tunnel: w1844 -> [w1869]
                  frame #0 {
                    n760 = Wait (ms)(milliseconds to wait=20) -> ()  [unwired: 1 out]
                  }
                }
                n761 = call-poly <vilib>:"Wait for Move Complete.flx"("Poll Interval (20 ms)"=5, "error in (no error)"=w1848, "Axis or Vector Space"=w1847, "Board ID"=w1845) -> ("error out"=w1855:errorcluster)  [unwired: 4 in, 3 out]
                n762 = property class="niScope"(reference=w1851, error in=w1855) -> (error out=w1838:errorcluster, "Records Done"=w1846:i32)  [unwired: 1 out]
                n763 = local write "Read Loop"(w1841) -> ()
                n764 = local read "stop out"() -> (w1852:bool)
                n765 = case shown="No Error" w1838 {
                  selector: w1838 -> [w1861 _]
                  tunnel: w1850 -> [w1867 _]
                  tunnel: [w1865 w1868] -> w1842
                  tunnel: w1839 -> [w1862 w1868]
                  frame No Error {
                    n766 = Lossy Enqueue Element(queue=w1862, element=w1867, error in (no error)=w1861) -> (queue out=w1866:refnum<queue>, error out=w1864:errorcluster)  [unwired: 2 out]
                    n767 = Get Queue Status(queue=w1866, error in (no error)=w1864) -> (queue out=w1865:refnum<queue>, # elements in queue=w1863:i32)  [unwired: 1 in, 6 out]
                    n768 = local write "Record queue"(w1863) -> ()
                  }
                  frame Error {
                  }
                }
                n769 = Not(x=w1854) -> (.not. x?=w1859:bool)
              }
              n770 = while {
                tunnel: w1742 -> [w1792]
                tunnel: w1734 -> [w1791]
                tunnel: w1740 -> [w1787]
                tunnel: w1741 -> [w1790]
                shift-right: [w1785] -> _
                shift-left: w1736 -> [w1786]
                tunnel: [w1784] -> _
                tunnel: w1739 -> [w1779]
                tunnel: i16[] [1, 1, 1, 1, 2, 2, 2, 2, 2, 2] -> [w1778]
                tunnel: 10 -> [w1777]
                tunnel: w1737 -> [w1776]
                tunnel: [w1774] -> w1733
                tunnel: w1730 -> [_]
                tunnel: [w1773] -> w1729
                i -> [w1788]
                stop <- w1789 stop-if-true
                n771 = local write "SF Index"(w1788) -> ()
                n772 = Dequeue Element(queue=w1792, timeout in ms (-1)=1000) -> (element=w1780:i8[][])  [unwired: 1 in, 3 out]
                n773 = Multiply(x=w1776, y=w1777) -> (x*y=w1781:i32)
                n774 = Reshape Array(w1780, w1791, w1781) -> (w1782:i8[][])
                n775 = for {
                  N: w1777 -> [_]
                  tunnel: w1779 -> [w1800]
                  tunnel: [w1803] -> w1783
                  tunnel: w1787 -> [w1802]
                  shift-right: [w1795] -> _
                  shift-left: w1782 -> [w1805]
                  tunnel: w1776 -> [w1794]
                  tunnel: w1778 -> [w1793] mode=indexing
                  i -> [w1801]
                  n776 = Index Array(array=w1800, index=w1801) -> (element=w1799:T11)
                  n777 = Delete From Array(array=w1805, length=w1794, index (col)=0 ("disabled index (col)")) -> (deleted portion=w1798:i8[], array with subset deleted=w1795:i8[][])  [unwired: 1 in]
                  n778 = for {
                    tunnel: w1798 -> [w1808] mode=indexing
                    tunnel: [w1807] -> w1797 mode=indexing
                    n779 = call-poly <vilib>:"Mean.vi"("X"=w1808) -> ("mean"=w1809:dbl)  [unwired: 1 out]
                    n780 = To Word Integer(number=w1809) -> (16bit integer=w1806:i16)
                    n781 = Subtract(x=w1808, y=w1806) -> (x-y=w1807:i16)
                  }
                  n782 = call-poly "TimeShiftDataPoly.vi"("output cluster"=w1799, "Array In"=w1797) -> ("Array Out"=w1804:i16[][])  [unwired: 2 in]
                  n783 = in-place {
                    in-place-border: w1804 -> [w1811]
                    in-place-border: w1793 -> [w1812]
                    n784 = in-place-dvr #15(w1802) -> (w1813:i16[][])  [unwired: 1 out]
                    n785 = case shown="2" w1812 {
                      selector: w1812 -> [_ w1816]
                      tunnel: w1811 -> [w1815 w1818]
                      tunnel: [w1815 w1817] -> w1810
                      frame 0, Default {
                      }
                      frame 2 {
                        n786 = Multiply(x=w1816, y=w1818) -> (x*y=w1817:i16[][])
                      }
                    }
                    n787 = Add(x=w1810, y=w1813) -> (x+y=w1814:i16[][])
                    n788 = in-place-dvr #15(w1814) -> (w1803:refnum<data-value>)  [unwired: 1 out]
                  }
                }
                n789 = local read "stop out"() -> (w1789:bool)
                n790 = in-place {
                  in-place-border: w1790 -> [w1823]
                  in-place-border: [w1819] -> w1774
                  n791 = in-place-dvr #16(w1783) -> (w1820:i16[][])  [unwired: 1 out]
                  n792 = Multiply(x=i16 0, y=w1820) -> (x*y=w1822:i16[][])
                  n793 = Enqueue Element(queue=w1823, element=w1820) -> (queue out=w1819:refnum<queue>)  [unwired: 2 in, 2 out]
                  n794 = in-place-dvr #16(w1822) -> (w1773:refnum<data-value>)  [unwired: 1 out]
                }
                n795 = Tick Count (ms)() -> (millisecond timer value=w1785:u32)
                n796 = Subtract(x=w1785, y=w1786) -> (x-y=w1784:u32)
              }
              n797 = while {
                tunnel: w1754 -> [w1833]
                tunnel: w1741 -> [w1829]
                tunnel: [w1831] -> w1753
                shift-right: [w1824] -> _
                shift-left: TRUE -> [w1825]
                tunnel: w1730 -> [_]
                i -> [w1834]
                stop <- w1831 stop-if-true
                # "Slightly faster version to read data"
                # "Get and display data"
                n798 = Dequeue Element(queue=w1829, timeout in ms (-1)=1000) -> (element=w1826:i16[][])  [unwired: 1 in, 3 out]
                n799 = case shown="True" w1825 {
                  tunnel: w1826 -> [w1835 w1837]
                  tunnel: [w1835 w1836] -> w1830
                  frame False {
                  }
                  frame True {
                    n800 = call "ReverseData.vi"("Array in"=w1837) -> ("Array out"=w1836:i16[][])
                  }
                }
                n801 = Not(x=w1825) -> (.not. x?=w1824:bool)
                n802 = Increment(x=w1834) -> (x+1=w1828:i32)
                n803 = local write "Display index"(w1828) -> ()
                n804 = call "CurrentPlane.vi"("bits A/D"=13, "Axis Vals"=w1833, "Frame"=w1828, "Data"=w1830) -> ("stop out"=w1831:bool)  [unwired: 6 in, 1 out]
                n805 = local write "stop out"(w1831) -> ()
              }
              n806 = node-c288(w1758) -> ()
              n807 = Compound Arithmetic op=AND(w1760, w1765, w1753) -> (w1750:bool)
              n808 = Release Queue(queue=w1764, force destroy? (F)=w1750) -> ()  [unwired: 1 in, 3 out]
              n809 = call <instrlib>:"niScope Abort.vi"("instrument handle"=w1731) -> ()  [unwired: 13 in, 2 out]
              n810 = Delete Data Value Reference(data value reference=w1729) -> ()  [unwired: 1 in, 2 out]
              n811 = Release Queue(queue=w1763, force destroy? (F)=w1750) -> ()  [unwired: 1 in, 3 out]
              n812 = Release Queue(queue=w1733, force destroy? (F)=w1750) -> ()  [unwired: 1 in, 3 out]
            }
            frame "Drop Ch 5 (3 Trig)" {
              w1925 = 2 ("index")
              w1950 = 5
              # "Reduced data case that drop ring 5 receive using rcv on 3,4,5"
              # "Restructure file names"
              # "Read queue and send to files. About same as reading channel by channel"
              n813 = Reshape Array(w1951, w1950, w1950) -> (w1923:T12)
              n814 = Index Array(array=w1912, index=0 ("length")) -> (element=w1911)
              n815 = Index Array(array=w1912, index=1) -> (element=w1914)
              n816 = Initialize Array(i16 0, w1917, w1922) -> (w1940:i16[][])
              n817 = Array Subset(array=w1923, index (row)=2 ("index"), index (col)=w1925, length (col)=w1925) -> (w1924:T12)  [unwired: 1 in]
              n818 = Array Subset(array=w1923, length (col)=2 ("index")) -> (w1927:T12)  [unwired: 3 in]
              n819 = Obtain Queue(max queue size (-1, unlimited)=6, element data type=T9 {"gain"=0.0, "wfm"=[], TRUE, "max queue size (-1, unlimited)"=15}) -> (queue out=w1953:refnum<queue>)  [unwired: 3 in, 2 out]
              n820 = New Data Value Reference(data value=w1940) -> (data value reference=w1939:refnum<data-value>)  [unwired: 1 in, 1 out]
              n821 = Reshape Array(w1927, 10) -> (w1926:T13)
              n822 = Reshape Array(w1924, 6) -> (w1937:T13)
              n823 = Obtain Queue(max queue size (-1, unlimited)=3, element data type=cluster{"gain":dbl, bool, "wfm":i16[][]} {"gain"=0.0, TRUE, "wfm"=[]}) -> (queue out=w1941:refnum<queue>)  [unwired: 3 in, 2 out]
              n824 = expression code="x*5"(w1917) -> (w1920:dbl)
              n825 = expression code="x*3"(w1917) -> (w1916:dbl)
              n826 = Tick Count (ms)() -> (millisecond timer value=w1934:u32)
              n827 = Build Array(w1926, w1937) -> (w1936:T12)
              n828 = while {
                tunnel: w1953 -> [w1973]
                tunnel: w1922 -> [w1972]
                tunnel: [w1968] -> w1945
                tunnel: w1917 -> [w1971]
                tunnel: w1939 -> [w1966]
                tunnel: w1941 -> [w1970]
                tunnel: w1936 -> [w1961]
                tunnel: i32[] [10, 6] -> [w1965]
                shift-right: [w1963] -> _
                shift-left: w1934 -> [w1964]
                tunnel: [w1962] -> _
                tunnel: 10000 -> [w1957]
                tunnel: i16[] [1, 1, 1, 1, 2, 2, 2, 2, 2, 2] -> [w1956]
                tunnel: [w1955] -> w1921
                i -> [w1967]
                stop <- w1968 stop-if-true
                n829 = for {
                  tunnel: w1972 -> [w1984]
                  tunnel: w1971 -> [w1995]
                  tunnel: w1973 -> [w1998]
                  tunnel: [w1994] -> w1960 mode=indexing
                  tunnel: [w1993] -> w1969
                  tunnel: [w1992] -> w1958
                  tunnel: w1966 -> [w1991]
                  tunnel: w1961 -> [_] mode=indexing
                  tunnel: w1965 -> [w1988]
                  tunnel: w1961 -> [w1990]
                  tunnel: w1957 -> [w1987]
                  tunnel: w1956 -> [w1983]
                  n830 = Dequeue Element(queue=w1998, timeout in ms (-1)=w1987) -> (element=w1997:T9)  [unwired: 1 in, 3 out]
                  n831 = Unbundle(w1997) -> ("gain"=w1993:dbl, "wfm"=w1996:i8[][], w1994:bool, "max queue size (-1, unlimited)"=w1985:i32)
                  n832 = Index Array(array=w1988, index=w1985) -> (element=w1986:i32)
                  n833 = Index Array(array=w1990, index (row)=w1985) -> (element=w1989:T13)  [unwired: 1 in]
                  n834 = Multiply(x=w1984, y=w1986) -> (x*y=w1982:i32)
                  n835 = Reshape Array(w1996, w1995, w1982) -> (w1981:i8[][])
                  n836 = for {
                    N: w1986 -> [_]
                    tunnel: w1989 -> [w2006]
                    tunnel: [w2009] -> w1992
                    tunnel: w1991 -> [w2008]
                    shift-right: [w1999] -> _
                    shift-left: w1981 -> [w2011]
                    tunnel: w1983 -> [w2001] mode=indexing
                    tunnel: w1984 -> [w2000]
                    i -> [w2007]
                    n837 = Index Array(array=w2006, index=w2007) -> (element=w2005:T11)
                    n838 = Delete From Array(array=w2011, length=w2000, index (col)=0 ("disabled index (col)")) -> (deleted portion=w2004:i8[], array with subset deleted=w1999:i8[][])  [unwired: 1 in]
                    n839 = for {
                      tunnel: w2004 -> [w2014] mode=indexing
                      tunnel: [w2013] -> w2003 mode=indexing
                      n840 = call-poly <vilib>:"Mean.vi"("X"=w2014) -> ("mean"=w2015:dbl)  [unwired: 1 out]
                      n841 = To Word Integer(number=w2015) -> (16bit integer=w2012:i16)
                      n842 = Subtract(x=w2014, y=w2012) -> (x-y=w2013:i16)
                    }
                    n843 = call-poly "TimeShiftDataPoly.vi"("output cluster"=w2005, "Array In"=w2003) -> ("Array Out"=w2010:i16[][])  [unwired: 2 in]
                    n844 = in-place {
                      in-place-border: w2010 -> [w2017]
                      in-place-border: w2001 -> [w2018]
                      n845 = in-place-dvr #17(w2008) -> (w2019:i16[][])  [unwired: 1 out]
                      n846 = case shown="2" w2018 {
                        selector: w2018 -> [_ w2022]
                        tunnel: w2017 -> [w2021 w2024]
                        tunnel: [w2021 w2023] -> w2016
                        frame 0, Default {
                        }
                        frame 2 {
                          n847 = Multiply(x=w2022, y=w2024) -> (x*y=w2023:i16[][])
                        }
                      }
                      n848 = Add(x=w2016, y=w2019) -> (x+y=w2020:i16[][])
                      n849 = in-place-dvr #17(w2020) -> (w2009:refnum<data-value>)  [unwired: 1 out]
                    }
                  }
                }
                n850 = local write "SF Index"(w1967) -> ()
                n851 = local read "stop out"() -> (w1968:bool)
                n852 = Or Array Elements(Boolean array=w1960) -> (logical OR=w1959:bool)
                n853 = in-place {
                  in-place-border: w1970 -> [w1980]
                  in-place-border: w1959 -> [w1979]
                  in-place-border: w1969 -> [w1978]
                  n854 = in-place-dvr #18(w1958) -> (w1974:i16[][])  [unwired: 1 out]
                  n855 = Bundle("gain"=w1978, w1979, w1974) -> (w1977:cluster{"gain":dbl, bool, i16[][]})  [unwired: 1 in]
                  n856 = Multiply(x=i16 0, y=w1974) -> (x*y=w1976:i16[][])
                  n857 = Enqueue Element(queue=w1980, element=w1977) -> ()  [unwired: 2 in, 3 out]
                  n858 = in-place-dvr #18(w1976) -> (w1955:refnum<data-value>)  [unwired: 1 out]
                }
                n859 = Tick Count (ms)() -> (millisecond timer value=w1963:u32)
                n860 = Subtract(x=w1963, y=w1964) -> (x-y=w1962:u32)
              }
              n861 = while {
                tunnel: w1943 -> [w2090]
                tunnel: w1941 -> [w2084]
                tunnel: [w2087] -> _
                tunnel: [w2089] -> w1944
                i -> [w2091]
                stop <- w2087 stop-if-true
                # "Slightly faster version to read data"
                # "Get and display data"
                n862 = Dequeue Element(queue=w2084, timeout in ms (-1)=5000) -> (queue out=w2089:refnum<queue>, element=w2086:cluster{"gain":dbl, bool, "wfm":i16[][]})  [unwired: 1 in, 2 out]
                n863 = Unbundle(w2086) -> ("gain"=w2081:dbl, w2082:bool, "wfm"=w2083:i16[][])
                n864 = case shown="False" w2082 {
                  tunnel: w2083 -> [w2092 w2094]
                  tunnel: [w2092 w2093] -> w2085
                  frame False {
                  }
                  frame True {
                    n865 = call "ReverseData.vi"("Array in"=w2094) -> ("Array out"=w2093:i16[][])
                  }
                }
                n866 = Increment(x=w2091) -> (x+1=w2080:i32)
                n867 = local write "Display index"(w2080) -> ()
                n868 = call "CurrentPlane.vi"("gain"=w2081, "bits A/D"=13, "Axis Vals"=w2090, "Frame"=w2080, "Data"=w2085) -> ("stop out"=w2087:bool)  [unwired: 5 in, 1 out]
                n869 = local write "stop out"(w2087) -> ()
              }
              n870 = global read "MotionGlobals.vi" "DigTimeOut"() -> (w1933)
              n871 = while {
                tunnel: w1911 -> [w2039]
                tunnel: w1953 -> [w2038]
                tunnel: w1914 -> [w2037]
                tunnel: w1922 -> [w2036]
                tunnel: [w2035] -> w1946
                tunnel: w1938 -> [w2033]
                shift-right: [w2031] -> _
                shift-left: w1934 -> [w2032]
                tunnel: [w2030] -> _
                tunnel: w1933 -> [w2029]
                tunnel: "0,1" -> [w2028]
                tunnel: w1920 -> [w2027]
                tunnel: w1916 -> [w2026]
                tunnel: 2 -> [w2025]
                stop <- w2034 stop-if-true
                n872 = for {
                  N: w2025 -> [_]
                  tunnel: w2036 -> [w2053]
                  tunnel: w2039 -> [w2055]
                  tunnel: w2028 -> [w2054]
                  tunnel: w2038 -> [w2052]
                  tunnel: [w2048] -> _
                  tunnel: w2037 -> [w2047]
                  tunnel: [w2045] -> w2035
                  tunnel: w2033 -> [w2044]
                  tunnel: w2029 -> [w2043]
                  tunnel: w2027 -> [w2041]
                  tunnel: w2026 -> [w2040]
                  i -> [w2042]
                  # "Read data"
                  n873 = case shown="0" w2042 {
                    tunnel: w2055 -> [w2061 w2070]
                    tunnel: w2054 -> [w2059 w2069]
                    tunnel: w2053 -> [w2062 w2075]
                    tunnel: [w2063 w2074] -> w2051
                    tunnel: [w2056 w2068] -> w2050
                    tunnel: [w2064 w2073] -> w2048
                    tunnel: w2047 -> [w2065 _]
                    tunnel: [w2060 _] -> w2046
                    tunnel: w2044 -> [w2058 _]
                    tunnel: w2043 -> [_ w2071]
                    tunnel: w2041 -> [_ _]
                    tunnel: w2040 -> [_ w2066]
                    frame 0 {
                      # "Read files and queue it up."
                      n874 = call <instrlib>:"niScope Initiate Acquisition.vi"("instrument handle"=w2065) -> ("error out"=w2057:errorcluster)  [unwired: 2 in, 12 out]
                      n875 = call "Rapid Read_NI.vi"("NI Card"=w2061, "Channel"=w2059, "Motion Board ID"=w2058, "rf points per line"=w2062, "error in"=w2057) -> ("dig gain"=w2063:dbl, "Array"=w2056:i8[][], "Reverse?"=w2060:bool, "error out"=w2064:errorcluster)  [unwired: 7 in]
                    }
                    frame 1, Default {
                      n876 = property class="niScope"(reference=w2070, "Fetch Record Number"=0 ("Fetch:Fetch Record Number"), "Fetch Number of Records"=w2066) -> (reference out=w2076:refnum<k15>, error out=w2072:errorcluster)  [unwired: 1 in]
                      n877 = call-poly <instrlib>:"niScope Fetch (poly).vi"("timeout"=w2071, "error in"=w2072, "numSamples"=w2075, "channels"=w2069, "instrument handle"=w2076) -> ("error out"=w2073:errorcluster, "wfm"=w2068:i8[][], "wfm info"=w2078:T14)  [unwired: 4 out]
                      n878 = Index Array(array=w2078) -> (element=w2077:T15)  [unwired: 1 in]
                      n879 = Unbundle By Name(w2077) -> ("gain"=w2074:dbl)
                    }
                  }
                  n880 = local write "Read Data index"(w2042) -> ()
                  n881 = Bundle("gain"=w2051, "wfm"=w2050, "Reverse?"=w2046, w2042) -> (w2049:T16)  [unwired: 1 in]
                  n882 = Enqueue Element(queue=w2052, element=w2049) -> (queue out=w2045:refnum<queue>)  [unwired: 2 in, 2 out]
                }
                n883 = local read "stop out"() -> (w2034:bool)
                n884 = Tick Count (ms)() -> (millisecond timer value=w2031:u32)
                n885 = Subtract(x=w2031, y=w2032) -> (x-y=w2030:u32)
              }
              n886 = Release Queue(queue=w1946, force destroy? (F)=w1945) -> ()  [unwired: 1 in, 3 out]
              n887 = Release Queue(queue=w1944, force destroy? (F)=w1945) -> ()  [unwired: 1 in, 3 out]
              n888 = Delete Data Value Reference(data value reference=w1921) -> ()  [unwired: 1 in, 2 out]
            }
          }
        }
      }
    }
    frame #6 {
      n889 = case shown="4, Default" w2095 {
        tunnel: w2097 -> [_ w2100]
        frame 1 {
        }
        frame 4, Default {
          n890 = for {
            tunnel: w2100 -> [w2103] mode=indexing
            n891 = call <vilib>:"DAQmx Stop Task.vi"("task/channels in"=w2103) -> ("task out"=w2102:refnum<k21>, "error out"=w2101:errorcluster)  [unwired: 13 in]
            n892 = call <vilib>:"DAQmx Clear Task.vi"("task in"=w2102, "error in"=w2101) -> ()  [unwired: 13 in, 1 out]
          }
        }
      }
      n893 = case shown="\"UHI Allen\", \"CUMC RT\"" w2099 {
        frame "Hawaii", Default {
          # "turn off real time trig"
          n894 = call-poly <vilib>:"DAQmx Write.vi"("task/channels in"=refnum<k21> "DIO-L2 L3", "data"=bool[] [TRUE, FALSE]) -> ()  [unwired: 11 in, 3 out]
        }
        frame "UHI Allen", "CUMC RT" {
        }
      }
      n895 = local write "stop out"(FALSE ("stop out")) -> ()
      n896 = local write "Save Raw"(FALSE ("Save Raw")) -> ()
    }
  }
  n897 = case shown="\"Full 25 Ch\", Default" w35 {
    tunnel: w39 -> [w2107 w2112]
    tunnel: w38 -> [_ w2111]
    tunnel: w37 -> [w2106 w2110]
    tunnel: [w2107 w2109] -> w20
    tunnel: [w2106 w2108] -> w19
    frame "1T/5R Deep Mem", "Line by line All" {
    }
    frame "Full 25 Ch", Default {
      n898 = call <vilib>:"Stop Program.flx"("error in (no error)"=w2110, "Program (1)"=w2111, "Board ID"=w2112) -> ("error out"=w2108:errorcluster, "Bd ID Out"=w2109:T2)  [unwired: 4 out]
    }
  }
  n899 = case shown="True" "return to start" {
    tunnel: w40 -> [_ w2120]
    tunnel: w36 -> [_ w2128]
    tunnel: w20 -> [w2114 w2119]
    tunnel: w19 -> [w2113 w2118]
    tunnel: [w2114 w2127] -> w18
    tunnel: w29 -> [_ w2126]
    tunnel: w28 -> [_ w2125]
    tunnel: [w2113 w2124] -> w27
    frame False {
    }
    frame True {
      n900 = call "MoveMotor.vi"("error in (no error)"=w2118, "Target Position (0)"=w2128, "Axis or Vector Space"=w2120, "Motion Bd ID"=w2119) -> ("error out"=w2116:errorcluster, "Resource Output"=w2115:u16, "Bd ID Out"=w2117:u8)  [unwired: 1 in, 4 out]
      n901 = call "Load Acceleration/Deceleration.flx"("Acceleration (100000)"=w2125, "error in (no error)"=w2116, "Axis or Vector Space"=w2115, "Board ID"=w2117) -> ("error out"=w2123:errorcluster, "Resource Output"=w2121:T18, "Bd ID Out"=w2122:T2)  [unwired: 1 in, 2 out]
      n902 = call <vilib>:"Load Velocity.flx"("Velocity (10000)"=w2126, "error in (no error)"=w2123, "Axis or Vector Space"=w2121, "Board ID"=w2122) -> ("error out"=w2124:errorcluster, "Bd ID Out"=w2127:T2)  [unwired: 4 out]
    }
  }
  "error out" <- w27
  n903 = flat-sequence {
    tunnel: w18 -> [w2129]
    frame #0 {
      "Bd ID Out" <- w2129
    }
    frame #1 {
      n904 = Wait (ms)(milliseconds to wait=u32 10) -> ()  [unwired: 1 out]
    }
  }
